vi "Synthetic_Jet_Per_Block.vi"() -> (5 "Plug in titles":string[](array[string]), 7 "Plug in values":string[](array[string]))   [LabVIEW 2011]
uses:
  Globals/Meas_global.vi
  Globals/Plug_in_data_global.vi
  Acquisition/Data_Translation/DataTranslation_global.vi
  <vilib>/Analysis/baseanly.llb/Scale 1D.vi
  <vilib>/Analysis/1siggen.llb/Ramp Pattern by Samples.vi
  <vilib>/Analysis/NI_AALBase.lvlib
panel:
  out "Pressure":cluster{dbl[], dbl[]}[](graph)=[{[0.0, 0.006711409395973154, 0.013422818791946308, 0.020134228187919462, 0.026845637583892617, 0.03355704697986577, 0.040268456375838924, 0.04697986577181208, 0.053691275167785234, 0.060402684563758385, 0.06711409395973154, 0.0738255033557047, 0.08053691275167785, 0.087248322147651, 0.09395973154362416, 0.10067114093959731, 0.10738255033557047, 0.11409395973154361, 0.12080536912751677, 0.12751677852348994, 0.1342281879194631, 0.14093959731543626, 0.1476510067114094, 0.15436241610738255, 0.1610738255033557, 0.16778523489932887, 0.174496644295302, 0.18120805369127518, 0.18791946308724833, 0.1946308724832215, 0.20134228187919462, 0.2080536912751678, 0.21476510067114093, 0.2214765100671141, 0.22818791946308722, 0.23489932885906042, 0.24161073825503354, 0.24832214765100674, 0.2550335570469799, 0.261744966442953, 0.2684563758389262, 0.2751677852348993, 0.2818791946308725, 0.2885906040268456, 0.2953020134228188, 0.30201342281879195, 0.3087248322147651, 0.31543624161073824, 0.3221476510067114, 0.3288590604026846, 0.33557046979865773, 0.3422818791946309, 0.348993288590604, 0.35570469798657717, 0.36241610738255037, 0.36912751677852346, 0.37583892617449666, 0.3825503355704698, 0.389261744966443, 0.3959731543624161, 0.40268456375838924, 0.40939597315436244, 0.4161073825503356, 0.4228187919463087, 0.42953020134228187, 0.436241610738255, 0.4429530201342282, 0.44966442953020136, 0.45637583892617445, 0.46308724832214765, 0.46979865771812085, 0.476510067114094, 0.4832214765100671, 0.4899328859060403, 0.4966442953020135, 0.5033557046979865, 0.5100671140939598, 0.5167785234899329, 0.523489932885906, 0.5302013422818792, 0.5369127516778524, 0.5436241610738255, 0.5503355704697986, 0.5570469798657718, 0.563758389261745, 0.5704697986577181, 0.5771812080536912, 0.5838926174496645, 0.5906040268456376, 0.5973154362416107, 0.6040268456375839, 0.610738255033557, 0.6174496644295302, 0.6241610738255033, 0.6308724832214765, 0.6375838926174497, 0.6442953020134228, 0.6510067114093959, 0.6577181208053692, 0.6644295302013422, 0.6711409395973155, 0.6778523489932886, 0.6845637583892618, 0.6912751677852349, 0.697986577181208, 0.7046979865771812, 0.7114093959731543, 0.7181208053691275, 0.7248322147651007, 0.7315436241610739, 0.7382550335570469, 0.7449664429530202, 0.7516778523489933, 0.7583892617449665, 0.7651006711409396, 0.7718120805369127, 0.778523489932886, 0.785234899328859, 0.7919463087248322, 0.7986577181208054, 0.8053691275167785, 0.8120805369127516, 0.8187919463087249, 0.825503355704698, 0.8322147651006712, 0.8389261744966443, 0.8456375838926175, 0.8523489932885906, 0.8590604026845637, 0.8657718120805369, 0.87248322147651, 0.8791946308724832, 0.8859060402684564, 0.8926174496644295, 0.8993288590604027, 0.9060402684563759, 0.9127516778523489, 0.9194630872483222, 0.9261744966442953, 0.9328859060402683, 0.9395973154362417, 0.9463087248322147, 0.953020134228188, 0.9597315436241611, 0.9664429530201342, 0.9731543624161074, 0.9798657718120806, 0.9865771812080536, 0.993288590604027, 1.0], [-0.25922546202362834, -0.4891204155324937, -0.6904080016618581, -0.8480493006444599, -0.9531546399067627, -0.9992739938596971, -0.9832658992629901, -0.9072023850623537, -0.7746259523585205, -0.5945933728335518, -0.3769969137121356, -0.13751047137392813, 0.11253663462306722, 0.35342670947288585, 0.5732288768268338, 0.7575057737083402, 0.8937918066214312, 0.975804049085562, 0.9976606124806482, 0.9561531939230075, 0.8553255918389477, 0.701995449856294, 0.5055203180524536, 0.2763271807993936, 0.030323873228706288, -0.21741726507064232, -0.4516233755794559, -0.6584586521118543, -0.8235859911563818, -0.9390514751472424, -0.9955643936504392, -0.9910192978985559, -0.924948310387722, -0.8008270925752599, -0.6293499874067777, -0.4169670204713452, -0.17941892779202917, 0.0689237672980099, 0.3128216261012807, 0.5372691486722271, 0.7283971090032636, 0.8738401730635315, 0.9660454611476949, 1.0, 0.9671483152639606, 0.8766808579084586, 0.7323072281427515, 0.5414132065636502, 0.3170325236361138, 0.0740370000188787, -0.17510777079208098, -0.41165326882024633, -0.6247046321897792, -0.7985879645210232, -0.9226089228683702, -0.9906182600380955, -0.9962662099062448, -0.9403548481937384, -0.826593775109834, -0.661900893747472, -0.4568702875871448, -0.22202920046593577, 0.02487644229078725, 0.27271784005525096, 0.5005073447966999, 0.6983526892904462, 0.8524849069940206, 0.954047745155591, 0.9966580178294975, 0.9763053464111373, 0.8967327509314734, 0.7603130387315623, 0.5771724157880267, 0.3585399421937547, 0.11718198984006566, -0.1316620025755488, -0.3727525963555975, -0.5900482770816685, -0.7717852675135934, -0.9053977146902825, -0.9835666776583354, -0.9990734749294669, -0.9541572345579136, -0.850889985489387, -0.6934157856153104, -0.4943673275401826, -0.26353661902357656, -0.017834089848234407, 0.23020782684645943, 0.4626092669832018, 0.6666372784923779, 0.8293249705524385, 0.9402453587914156, 0.993449714945815, 0.9842592639769333, 0.9139439591095612, 0.7875167735994525, 0.6119290303612525, 0.39834294984443913, 0.1592909651883969, -0.08865069204118191, -0.33274906977468277, -0.5549908841130975, -0.7432781595992073, -0.8855463405974977, -0.9741088681158134, -1.001914159774394, -0.9662217901934275, -0.8727465488844732, -0.723961502653703, -0.5304273151599044, -0.3054450754416776, -0.061246438243061585, 0.1873970352423227, 0.4244438305960635, 0.6338858532214537, 0.8049619205294755, 0.9253401183109746, 0.9892053975892771, 0.9910100679613483, 0.9305870303186635, 0.8139184327464221, 0.6452820124228671, 0.437343881774203, 0.20230227572276377, -0.045539122041699936, -0.2912416512170421, -0.519131415423606, -0.7137684570336703, -0.8649931502489075, -0.9626124494492849, -0.9992739938596971, -0.9772169115343806, -0.8929989608377183, -0.7531704268238946, -0.5669886001052015, -0.3462506777435128, -0.10325515412627774, 0.1451878004288764, 0.38474108241049404, 0.600633130624954, 0.7786605208476208, 0.9084965281716421, 0.9817527773490564, 0.9950538663876562, 0.9455925302642196, 0.83818122330427, 0.6770976826860506, 0.4746069829753056, 0.24411047267574976]}, {[0.0, 0.006711409395973154, 0.013422818791946308, 0.020134228187919462, 0.026845637583892617, 0.03355704697986577, 0.040268456375838924, 0.04697986577181208, 0.053691275167785234, 0.060402684563758385, 0.06711409395973154, 0.0738255033557047, 0.08053691275167785, 0.087248322147651, 0.09395973154362416, 0.10067114093959731, 0.10738255033557047, 0.11409395973154361, 0.12080536912751677, 0.12751677852348994, 0.1342281879194631, 0.14093959731543626, 0.1476510067114094, 0.15436241610738255, 0.1610738255033557, 0.16778523489932887, 0.174496644295302, 0.18120805369127518, 0.18791946308724833, 0.1946308724832215, 0.20134228187919462, 0.2080536912751678, 0.21476510067114093, 0.2214765100671141, 0.22818791946308722, 0.23489932885906042, 0.24161073825503354, 0.24832214765100674, 0.2550335570469799, 0.261744966442953, 0.2684563758389262, 0.2751677852348993, 0.2818791946308725, 0.2885906040268456, 0.2953020134228188, 0.30201342281879195, 0.3087248322147651, 0.31543624161073824, 0.3221476510067114, 0.3288590604026846, 0.33557046979865773, 0.3422818791946309, 0.348993288590604, 0.35570469798657717, 0.36241610738255037, 0.36912751677852346, 0.37583892617449666, 0.3825503355704698, 0.389261744966443, 0.3959731543624161, 0.40268456375838924, 0.40939597315436244, 0.4161073825503356, 0.4228187919463087, 0.42953020134228187, 0.436241610738255, 0.4429530201342282, 0.44966442953020136, 0.45637583892617445, 0.46308724832214765, 0.46979865771812085, 0.476510067114094, 0.4832214765100671, 0.4899328859060403, 0.4966442953020135, 0.5033557046979865, 0.5100671140939598, 0.5167785234899329, 0.523489932885906, 0.5302013422818792, 0.5369127516778524, 0.5436241610738255, 0.5503355704697986, 0.5570469798657718, 0.563758389261745, 0.5704697986577181, 0.5771812080536912, 0.5838926174496645, 0.5906040268456376, 0.5973154362416107, 0.6040268456375839, 0.610738255033557, 0.6174496644295302, 0.6241610738255033, 0.6308724832214765, 0.6375838926174497, 0.6442953020134228, 0.6510067114093959, 0.6577181208053692, 0.6644295302013422, 0.6711409395973155, 0.6778523489932886, 0.6845637583892618, 0.6912751677852349, 0.697986577181208, 0.7046979865771812, 0.7114093959731543, 0.7181208053691275, 0.7248322147651007, 0.7315436241610739, 0.7382550335570469, 0.7449664429530202, 0.7516778523489933, 0.7583892617449665, 0.7651006711409396, 0.7718120805369127, 0.778523489932886, 0.785234899328859, 0.7919463087248322, 0.7986577181208054, 0.8053691275167785, 0.8120805369127516, 0.8187919463087249, 0.825503355704698, 0.8322147651006712, 0.8389261744966443, 0.8456375838926175, 0.8523489932885906, 0.8590604026845637, 0.8657718120805369, 0.87248322147651, 0.8791946308724832, 0.8859060402684564, 0.8926174496644295, 0.8993288590604027, 0.9060402684563759, 0.9127516778523489, 0.9194630872483222, 0.9261744966442953, 0.9328859060402683, 0.9395973154362417, 0.9463087248322147, 0.953020134228188, 0.9597315436241611, 0.9664429530201342, 0.9731543624161074, 0.9798657718120806, 0.9865771812080536, 0.993288590604027, 1.0], [-0.06773154569815733, -0.3291387513527619, -0.5307198363636499, -0.7291484496532293, -0.8614105778258978, -0.9527614156827031, -1.0031655421930694, -0.9559138874040123, -0.8708679929898244, -0.7228435062106116, -0.5432943022183092, -0.27873462484239575, -0.09606837015936108, 0.17794872238047915, 0.4047141601312622, 0.6094477168634593, 0.7858444491344526, 0.8960746962885352, 0.9181065773071212, 0.9559008169322516, 0.9149541055858121, 0.7984189149891117, 0.6094477168634593, 0.4362388773443514, 0.2062855468416829, -0.026784834351717905, -0.25670274382380986, -0.4929255967385195, -0.6945066817494077, -0.8488361119712386, -0.9464564722400853, -1.0000130704717607, -0.9716408249799802, -0.9086622326149552, -0.7196910344893026, -0.5432943022183092, -0.3606280475352745, -0.11810025117794698, 0.127544595870113, 0.3700723922274406, 0.5874158358448734, 0.7826919774131437, 0.8866172811246085, 0.8740073942393727, 0.9685107038174874, 0.9307164641923568, 0.8078763301530385, 0.6818837243924114, 0.48660758282414107, 0.24407978646681344, 0.014161876994721509, -0.25039780038119197, -0.48031570985328387, -0.6724393797002453, -0.8299212816433852, -0.9275770629428083, -0.9874031835865249, -0.9905556553078338, -0.902357289172337, -0.7858220985756368, -0.5779714911527072, -0.38265992855386044, -0.12755766634187377, 0.039381650765192844, 0.33227815260231003, 0.5527740679410517, 0.7165254922962327, 0.8771598659606816, 0.9307164641923568, 1.0, 0.9338689359136656, 0.8519755132207868, 0.6944936112776469, 0.5023699414306856, 0.27245203195859363, 0.03622917904388393, -0.18111426457354876, -0.44252147022815336, -0.625187724911188, -0.7921270420182547, -0.8803254081537512, -0.9968605987504516, -0.9874031835865249, -0.8928998740084104, -0.7921270420182547, -0.625187724911188, -0.44567394194946225, -0.19684120214951692, 0.03622917904388393, 0.2944839129771795, 0.5180968790066537, 0.7039510264415737, 0.8614329283847134, 0.9464788227989014, 0.9622057603748693, 0.9716631755387962, 0.8677378718273314, 0.7259829074601595, 0.5275542941705804, 0.3385830960449279, 0.0866333055542501, -0.1558944908030775, -0.39211734371778717, -0.6063083156139111, -0.7795171551330188, -0.8897828233176781, -0.9433040005187766, -0.9968605987504516, -0.9275770629428083, -0.8299212816433852, -0.7102336193253758, -0.45513135711338903, -0.2126035607560615, 0.014161876994721509, 0.2503847299094312, 0.49291252626675885, 0.6724617302590611, 0.823638688759583, 0.9086491621431942, 0.9622057603748693, 0.9716631755387962, 0.8771598659606816, 0.7637771470852902, 0.5748059489596377, 0.3511929829301636, 0.10236024313021819, -0.11494777945663807, -0.3165288644675262, -0.5716665477100895, -0.7417229155078886, -0.8928998740084104, -1.0220449514903465, -0.9905556553078338, -0.9401515287974678, -0.8393786968073119, -0.7196910344893026, -0.5086525343144875, -0.3070714493035994, -0.03305435676375923, 0.20001602442964156, 0.4267814621804246, 0.6566993716525166, 0.8015713867104207, 0.9149541055858121, 0.9622057603748693, 0.9590532886535604, 0.8834648094032994, 0.8110288018743474, 0.634632069603354, 0.4047141601312622]}, {[0.0, 0.006711409395973154, 0.013422818791946308, 0.020134228187919462, 0.026845637583892617, 0.03355704697986577, 0.040268456375838924, 0.04697986577181208, 0.053691275167785234, 0.060402684563758385, 0.06711409395973154, 0.0738255033557047, 0.08053691275167785, 0.087248322147651, 0.09395973154362416, 0.10067114093959731, 0.10738255033557047, 0.11409395973154361, 0.12080536912751677, 0.12751677852348994, 0.1342281879194631, 0.14093959731543626, 0.1476510067114094, 0.15436241610738255, 0.1610738255033557, 0.16778523489932887, 0.174496644295302, 0.18120805369127518, 0.18791946308724833, 0.1946308724832215, 0.20134228187919462, 0.2080536912751678, 0.21476510067114093, 0.2214765100671141, 0.22818791946308722, 0.23489932885906042, 0.24161073825503354, 0.24832214765100674, 0.2550335570469799, 0.261744966442953, 0.2684563758389262, 0.2751677852348993, 0.2818791946308725, 0.2885906040268456, 0.2953020134228188, 0.30201342281879195, 0.3087248322147651, 0.31543624161073824, 0.3221476510067114, 0.3288590604026846, 0.33557046979865773, 0.3422818791946309, 0.348993288590604, 0.35570469798657717, 0.36241610738255037, 0.36912751677852346, 0.37583892617449666, 0.3825503355704698, 0.389261744966443, 0.3959731543624161, 0.40268456375838924, 0.40939597315436244, 0.4161073825503356, 0.4228187919463087, 0.42953020134228187, 0.436241610738255, 0.4429530201342282, 0.44966442953020136, 0.45637583892617445, 0.46308724832214765, 0.46979865771812085, 0.476510067114094, 0.4832214765100671, 0.4899328859060403, 0.4966442953020135, 0.5033557046979865, 0.5100671140939598, 0.5167785234899329, 0.523489932885906, 0.5302013422818792, 0.5369127516778524, 0.5436241610738255, 0.5503355704697986, 0.5570469798657718, 0.563758389261745, 0.5704697986577181, 0.5771812080536912, 0.5838926174496645, 0.5906040268456376, 0.5973154362416107, 0.6040268456375839, 0.610738255033557, 0.6174496644295302, 0.6241610738255033, 0.6308724832214765, 0.6375838926174497, 0.6442953020134228, 0.6510067114093959, 0.6577181208053692, 0.6644295302013422, 0.6711409395973155, 0.6778523489932886, 0.6845637583892618, 0.6912751677852349, 0.697986577181208, 0.7046979865771812, 0.7114093959731543, 0.7181208053691275, 0.7248322147651007, 0.7315436241610739, 0.7382550335570469, 0.7449664429530202, 0.7516778523489933, 0.7583892617449665, 0.7651006711409396, 0.7718120805369127, 0.778523489932886, 0.785234899328859, 0.7919463087248322, 0.7986577181208054, 0.8053691275167785, 0.8120805369127516, 0.8187919463087249, 0.825503355704698, 0.8322147651006712, 0.8389261744966443, 0.8456375838926175, 0.8523489932885906, 0.8590604026845637, 0.8657718120805369, 0.87248322147651, 0.8791946308724832, 0.8859060402684564, 0.8926174496644295, 0.8993288590604027, 0.9060402684563759, 0.9127516778523489, 0.9194630872483222, 0.9261744966442953, 0.9328859060402683, 0.9395973154362417, 0.9463087248322147, 0.953020134228188, 0.9597315436241611, 0.9664429530201342, 0.9731543624161074, 0.9798657718120806, 0.9865771812080536, 0.993288590604027, 1.0], [0.6373944760416457, 0.4107366158530138, 0.2092853682298436, -0.019859544398579457, -0.25407938835685134, -0.4807036397287289, -0.6620232061162826, -0.7980044787027606, -0.9012507637708912, -0.9264573763363528, -0.8937223888180068, -0.7829141199802374, -0.6771471736555602, -0.4781829784721823, -0.2641620333830344, -0.04758681822058906, 0.20172338446020602, 0.4157779383661059, 0.5794528759578378, 0.7658137648584848, 0.8967537149318688, 0.9521746537591312, 0.9496539925025853, 0.9118776824711464, 0.7985487523768298, 0.6499641735076223, 0.4560749096540908, 0.234458371978551, -0.002248524419510842, -0.23643475956102716, -0.4479686522103816, -0.6418915248806674, -0.7854347812367828, -0.8886810663049135, -0.8987301025143457, -0.8886810663049135, -0.82821880496456, -0.6871962098649912, -0.5109179659905284, -0.30442539585426615, -0.09037084194836505, 0.1664677356853132, 0.37548096707812095, 0.5265862072038764, 0.758251781088846, 0.8741013724397081, 0.9521746537591312, 0.9823889800209313, 0.9420920087329465, 0.816193381172654, 0.6927818060521538, 0.47620659088970607, 0.2747553432665359, 0.04308976938156619, -0.20117911078613437, -0.41019234217894335, -0.6015945535926824, -0.772831474954052, -0.8710364375090905, -0.9113334087970765, -0.8659951149959983, -0.8256981437080146, -0.6897168711215368, -0.5663389048177897, -0.3271113471631813, -0.11557745451382682, 0.11864238944444272, 0.34526664081632147, 0.5467178884394917, 0.7431614223663229, 0.8564567436438846, 0.9647443512251084, 0.9773476575078393, 0.9496539925025853, 0.8564567436438846, 0.702864451078338, 0.534148190973514, 0.3200936370676141, 0.10099776064861972, -0.14075045826253538, -0.3447223671422511, -0.5739008885874285, -0.7325345036660671, -0.8332601274776522, -0.8962094412577991, -0.8861604050483679, -0.8534254175300219, -0.7325345036660671, -0.5915119085664983, -0.3799780159171427, -0.16088213949815067, 0.08839445436589002, 0.32513495958070504, 0.5316275297169674, 0.7053851123348835, 0.8690600499266155, 0.9446126699894919, 0.9723063349947466, 0.9370506862198538, 0.8741013724397081, 0.7179548098008612, 0.5643625172353147, 0.3578699470990524, 0.10603908316171302, -0.12562649072325785, -0.3296320084197279, -0.5235212722732593, -0.7426171486922525, -0.82821880496456, -0.9239367150798062, -0.9339857512892373, -0.8659951149959983, -0.7602281686713211, -0.6217262348282977, -0.440406668440744, -0.20369977204268103, 0.02292447932919654, 0.26719335949689715, 0.4736859296331594, 0.657526157277261, 0.8388457236648147, 0.9118776824711464, 0.9723063349947466, 0.9672650124816545, 0.8892253399789851, 0.7658137648584848, 0.607180149779845, 0.4283812446488379, 0.1614264131722199, -0.07023916071274978, -0.30946671836735823, -0.54617361476542, -0.6746265123990136, -0.8206904300116756, -0.8937223888180068, -0.9289780375928997, -0.8811190825352758, -0.8030458012158527, -0.6368502023675753, -0.4656132810062046, -0.24903806584375807, -0.014851830702241725, 0.22689638820891336, 0.4409509421148133, 0.6323531535285536, 0.7960280911202844, 0.9068363599580538, 0.9849096412774775, 1.0, 0.9068363599580538]}]
  out "Displacement":cluster{dbl[], dbl[]}[](graph)=[{[0.0, 0.006711409395973154, 0.013422818791946308, 0.020134228187919462, 0.026845637583892617, 0.03355704697986577, 0.040268456375838924, 0.04697986577181208, 0.053691275167785234, 0.060402684563758385, 0.06711409395973154, 0.0738255033557047, 0.08053691275167785, 0.087248322147651, 0.09395973154362416, 0.10067114093959731, 0.10738255033557047, 0.11409395973154361, 0.12080536912751677, 0.12751677852348994, 0.1342281879194631, 0.14093959731543626, 0.1476510067114094, 0.15436241610738255, 0.1610738255033557, 0.16778523489932887, 0.174496644295302, 0.18120805369127518, 0.18791946308724833, 0.1946308724832215, 0.20134228187919462, 0.2080536912751678, 0.21476510067114093, 0.2214765100671141, 0.22818791946308722, 0.23489932885906042, 0.24161073825503354, 0.24832214765100674, 0.2550335570469799, 0.261744966442953, 0.2684563758389262, 0.2751677852348993, 0.2818791946308725, 0.2885906040268456, 0.2953020134228188, 0.30201342281879195, 0.3087248322147651, 0.31543624161073824, 0.3221476510067114, 0.3288590604026846, 0.33557046979865773, 0.3422818791946309, 0.348993288590604, 0.35570469798657717, 0.36241610738255037, 0.36912751677852346, 0.37583892617449666, 0.3825503355704698, 0.389261744966443, 0.3959731543624161, 0.40268456375838924, 0.40939597315436244, 0.4161073825503356, 0.4228187919463087, 0.42953020134228187, 0.436241610738255, 0.4429530201342282, 0.44966442953020136, 0.45637583892617445, 0.46308724832214765, 0.46979865771812085, 0.476510067114094, 0.4832214765100671, 0.4899328859060403, 0.4966442953020135, 0.5033557046979865, 0.5100671140939598, 0.5167785234899329, 0.523489932885906, 0.5302013422818792, 0.5369127516778524, 0.5436241610738255, 0.5503355704697986, 0.5570469798657718, 0.563758389261745, 0.5704697986577181, 0.5771812080536912, 0.5838926174496645, 0.5906040268456376, 0.5973154362416107, 0.6040268456375839, 0.610738255033557, 0.6174496644295302, 0.6241610738255033, 0.6308724832214765, 0.6375838926174497, 0.6442953020134228, 0.6510067114093959, 0.6577181208053692, 0.6644295302013422, 0.6711409395973155, 0.6778523489932886, 0.6845637583892618, 0.6912751677852349, 0.697986577181208, 0.7046979865771812, 0.7114093959731543, 0.7181208053691275, 0.7248322147651007, 0.7315436241610739, 0.7382550335570469, 0.7449664429530202, 0.7516778523489933, 0.7583892617449665, 0.7651006711409396, 0.7718120805369127, 0.778523489932886, 0.785234899328859, 0.7919463087248322, 0.7986577181208054, 0.8053691275167785, 0.8120805369127516, 0.8187919463087249, 0.825503355704698, 0.8322147651006712, 0.8389261744966443, 0.8456375838926175, 0.8523489932885906, 0.8590604026845637, 0.8657718120805369, 0.87248322147651, 0.8791946308724832, 0.8859060402684564, 0.8926174496644295, 0.8993288590604027, 0.9060402684563759, 0.9127516778523489, 0.9194630872483222, 0.9261744966442953, 0.9328859060402683, 0.9395973154362417, 0.9463087248322147, 0.953020134228188, 0.9597315436241611, 0.9664429530201342, 0.9731543624161074, 0.9798657718120806, 0.9865771812080536, 0.993288590604027, 1.0], [-0.25922546202362834, -0.4891204155324937, -0.6904080016618581, -0.8480493006444599, -0.9531546399067627, -0.9992739938596971, -0.9832658992629901, -0.9072023850623537, -0.7746259523585205, -0.5945933728335518, -0.3769969137121356, -0.13751047137392813, 0.11253663462306722, 0.35342670947288585, 0.5732288768268338, 0.7575057737083402, 0.8937918066214312, 0.975804049085562, 0.9976606124806482, 0.9561531939230075, 0.8553255918389477, 0.701995449856294, 0.5055203180524536, 0.2763271807993936, 0.030323873228706288, -0.21741726507064232, -0.4516233755794559, -0.6584586521118543, -0.8235859911563818, -0.9390514751472424, -0.9955643936504392, -0.9910192978985559, -0.924948310387722, -0.8008270925752599, -0.6293499874067777, -0.4169670204713452, -0.17941892779202917, 0.0689237672980099, 0.3128216261012807, 0.5372691486722271, 0.7283971090032636, 0.8738401730635315, 0.9660454611476949, 1.0, 0.9671483152639606, 0.8766808579084586, 0.7323072281427515, 0.5414132065636502, 0.3170325236361138, 0.0740370000188787, -0.17510777079208098, -0.41165326882024633, -0.6247046321897792, -0.7985879645210232, -0.9226089228683702, -0.9906182600380955, -0.9962662099062448, -0.9403548481937384, -0.826593775109834, -0.661900893747472, -0.4568702875871448, -0.22202920046593577, 0.02487644229078725, 0.27271784005525096, 0.5005073447966999, 0.6983526892904462, 0.8524849069940206, 0.954047745155591, 0.9966580178294975, 0.9763053464111373, 0.8967327509314734, 0.7603130387315623, 0.5771724157880267, 0.3585399421937547, 0.11718198984006566, -0.1316620025755488, -0.3727525963555975, -0.5900482770816685, -0.7717852675135934, -0.9053977146902825, -0.9835666776583354, -0.9990734749294669, -0.9541572345579136, -0.850889985489387, -0.6934157856153104, -0.4943673275401826, -0.26353661902357656, -0.017834089848234407, 0.23020782684645943, 0.4626092669832018, 0.6666372784923779, 0.8293249705524385, 0.9402453587914156, 0.993449714945815, 0.9842592639769333, 0.9139439591095612, 0.7875167735994525, 0.6119290303612525, 0.39834294984443913, 0.1592909651883969, -0.08865069204118191, -0.33274906977468277, -0.5549908841130975, -0.7432781595992073, -0.8855463405974977, -0.9741088681158134, -1.001914159774394, -0.9662217901934275, -0.8727465488844732, -0.723961502653703, -0.5304273151599044, -0.3054450754416776, -0.061246438243061585, 0.1873970352423227, 0.4244438305960635, 0.6338858532214537, 0.8049619205294755, 0.9253401183109746, 0.9892053975892771, 0.9910100679613483, 0.9305870303186635, 0.8139184327464221, 0.6452820124228671, 0.437343881774203, 0.20230227572276377, -0.045539122041699936, -0.2912416512170421, -0.519131415423606, -0.7137684570336703, -0.8649931502489075, -0.9626124494492849, -0.9992739938596971, -0.9772169115343806, -0.8929989608377183, -0.7531704268238946, -0.5669886001052015, -0.3462506777435128, -0.10325515412627774, 0.1451878004288764, 0.38474108241049404, 0.600633130624954, 0.7786605208476208, 0.9084965281716421, 0.9817527773490564, 0.9950538663876562, 0.9455925302642196, 0.83818122330427, 0.6770976826860506, 0.4746069829753056, 0.24411047267574976]}, {[0.0, 0.006711409395973154, 0.013422818791946308, 0.020134228187919462, 0.026845637583892617, 0.03355704697986577, 0.040268456375838924, 0.04697986577181208, 0.053691275167785234, 0.060402684563758385, 0.06711409395973154, 0.0738255033557047, 0.08053691275167785, 0.087248322147651, 0.09395973154362416, 0.10067114093959731, 0.10738255033557047, 0.11409395973154361, 0.12080536912751677, 0.12751677852348994, 0.1342281879194631, 0.14093959731543626, 0.1476510067114094, 0.15436241610738255, 0.1610738255033557, 0.16778523489932887, 0.174496644295302, 0.18120805369127518, 0.18791946308724833, 0.1946308724832215, 0.20134228187919462, 0.2080536912751678, 0.21476510067114093, 0.2214765100671141, 0.22818791946308722, 0.23489932885906042, 0.24161073825503354, 0.24832214765100674, 0.2550335570469799, 0.261744966442953, 0.2684563758389262, 0.2751677852348993, 0.2818791946308725, 0.2885906040268456, 0.2953020134228188, 0.30201342281879195, 0.3087248322147651, 0.31543624161073824, 0.3221476510067114, 0.3288590604026846, 0.33557046979865773, 0.3422818791946309, 0.348993288590604, 0.35570469798657717, 0.36241610738255037, 0.36912751677852346, 0.37583892617449666, 0.3825503355704698, 0.389261744966443, 0.3959731543624161, 0.40268456375838924, 0.40939597315436244, 0.4161073825503356, 0.4228187919463087, 0.42953020134228187, 0.436241610738255, 0.4429530201342282, 0.44966442953020136, 0.45637583892617445, 0.46308724832214765, 0.46979865771812085, 0.476510067114094, 0.4832214765100671, 0.4899328859060403, 0.4966442953020135, 0.5033557046979865, 0.5100671140939598, 0.5167785234899329, 0.523489932885906, 0.5302013422818792, 0.5369127516778524, 0.5436241610738255, 0.5503355704697986, 0.5570469798657718, 0.563758389261745, 0.5704697986577181, 0.5771812080536912, 0.5838926174496645, 0.5906040268456376, 0.5973154362416107, 0.6040268456375839, 0.610738255033557, 0.6174496644295302, 0.6241610738255033, 0.6308724832214765, 0.6375838926174497, 0.6442953020134228, 0.6510067114093959, 0.6577181208053692, 0.6644295302013422, 0.6711409395973155, 0.6778523489932886, 0.6845637583892618, 0.6912751677852349, 0.697986577181208, 0.7046979865771812, 0.7114093959731543, 0.7181208053691275, 0.7248322147651007, 0.7315436241610739, 0.7382550335570469, 0.7449664429530202, 0.7516778523489933, 0.7583892617449665, 0.7651006711409396, 0.7718120805369127, 0.778523489932886, 0.785234899328859, 0.7919463087248322, 0.7986577181208054, 0.8053691275167785, 0.8120805369127516, 0.8187919463087249, 0.825503355704698, 0.8322147651006712, 0.8389261744966443, 0.8456375838926175, 0.8523489932885906, 0.8590604026845637, 0.8657718120805369, 0.87248322147651, 0.8791946308724832, 0.8859060402684564, 0.8926174496644295, 0.8993288590604027, 0.9060402684563759, 0.9127516778523489, 0.9194630872483222, 0.9261744966442953, 0.9328859060402683, 0.9395973154362417, 0.9463087248322147, 0.953020134228188, 0.9597315436241611, 0.9664429530201342, 0.9731543624161074, 0.9798657718120806, 0.9865771812080536, 0.993288590604027, 1.0], [-1.8900299638896667, -0.3337772428099433, -1.6677337567546753, -1.445437549619689, -1.3342894460521906, -1.1118139677824157, -1.3342894460521906, -2.5569185852946408, -1.6677337567546753, -3.6683996209695926, -3.4461034138346065, -4.780059927779338, -4.224319409941858, -5.113504238481823, -5.558096652751805, -4.557763720644347, -5.891540963454291, -4.335467513509355, -2.668066688862134, -4.1131713063743645, -3.3349553102671083, -3.4461034138346065, -2.5569185852946408, -2.5569185852946408, -1.7788818603221734, -2.4457704817271475, -0.8895177606474244, -1.1118139677824157, -1.2231413424846975, -1.445437549619689, -2.0011780674571646, -0.8895177606474244, -3.4461034138346065, -1.8900299638896667, -3.890695828104584, -4.66891182421184, -4.1131713063743645, -4.335467513509355, -4.891208031346832, -5.446948549184308, -5.002356134914325, -5.780392859886797, -4.557763720644347, -1.6677337567546753, -4.557763720644347, -3.5572515174020998, -4.446615617076849, -2.5569185852946408, -3.5572515174020998, -1.7788818603221734, -1.8900299638896667, -0.667221553512433, -0.4449253463774415, -1.445437549619689, -0.667221553512433, -2.3346223781596493, -1.8900299638896667, -1.556585653187182, -3.0015109995646236, -3.112659103132117, -4.780059927779338, -4.891208031346832, -6.1138371705892816, -3.0015109995646236, -4.1131713063743645, -5.224652342049316, -5.558096652751805, -5.224652342049316, -4.446615617076849, -5.446948549184308, -2.8903628959971255, -4.002023202806866, -3.5572515174020998, -1.6677337567546753, -2.0011780674571646, -1.6677337567546753, -1.556585653187182, -0.22262913924245015, -1.7788818603221734, -1.1118139677824157, -2.4457704817271475, -1.556585653187182, -1.8900299638896667, -3.3349553102671083, -2.4457704817271475, -4.891208031346832, -3.223807206699615, -5.002356134914325, -4.557763720644347, -5.335800445616814, -5.891540963454291, -5.113504238481823, -6.1138371705892816, -4.1131713063743645, -4.780059927779338, -5.224652342049316, -3.3349553102671083, -2.779214792429632, -2.3346223781596493, -2.112326171024658, -0.8895177606474244, -2.0011780674571646, -1.445437549619689, -0.8895177606474244, -0.8895177606474244, -1.8900299638896667, -2.668066688862134, -0.5560734499449347, -3.6683996209695926, -2.5569185852946408, -1.2231413424846975, -5.335800445616814, -5.002356134914325, -4.780059927779338, -4.446615617076849, -5.558096652751805, -5.002356134914325, -5.335800445616814, -4.557763720644347, -3.890695828104584, -5.002356134914325, -3.223807206699615, -4.002023202806866, -2.4457704817271475, -2.112326171024658, -1.3342894460521906, -1.445437549619689, -2.112326171024658, -1.0006658642149175, -1.1118139677824157, -0.667221553512433, 1.0, -2.4457704817271475, -1.8900299638896667, -3.4461034138346065, -2.8903628959971255, -3.5572515174020998, -3.890695828104584, -5.224652342049316, -4.446615617076849, -4.1131713063743645, -5.558096652751805, -4.780059927779338, -5.446948549184308, -4.335467513509355, -5.002356134914325, -2.5569185852946408, -4.335467513509355, -5.558096652751805, -1.7788818603221734]}]
  out "Hot Wire":cluster{dbl[], dbl[]}[](graph)=[{[0.0, 0.006711409395973154, 0.013422818791946308, 0.020134228187919462, 0.026845637583892617, 0.03355704697986577, 0.040268456375838924, 0.04697986577181208, 0.053691275167785234, 0.060402684563758385, 0.06711409395973154, 0.0738255033557047, 0.08053691275167785, 0.087248322147651, 0.09395973154362416, 0.10067114093959731, 0.10738255033557047, 0.11409395973154361, 0.12080536912751677, 0.12751677852348994, 0.1342281879194631, 0.14093959731543626, 0.1476510067114094, 0.15436241610738255, 0.1610738255033557, 0.16778523489932887, 0.174496644295302, 0.18120805369127518, 0.18791946308724833, 0.1946308724832215, 0.20134228187919462, 0.2080536912751678, 0.21476510067114093, 0.2214765100671141, 0.22818791946308722, 0.23489932885906042, 0.24161073825503354, 0.24832214765100674, 0.2550335570469799, 0.261744966442953, 0.2684563758389262, 0.2751677852348993, 0.2818791946308725, 0.2885906040268456, 0.2953020134228188, 0.30201342281879195, 0.3087248322147651, 0.31543624161073824, 0.3221476510067114, 0.3288590604026846, 0.33557046979865773, 0.3422818791946309, 0.348993288590604, 0.35570469798657717, 0.36241610738255037, 0.36912751677852346, 0.37583892617449666, 0.3825503355704698, 0.389261744966443, 0.3959731543624161, 0.40268456375838924, 0.40939597315436244, 0.4161073825503356, 0.4228187919463087, 0.42953020134228187, 0.436241610738255, 0.4429530201342282, 0.44966442953020136, 0.45637583892617445, 0.46308724832214765, 0.46979865771812085, 0.476510067114094, 0.4832214765100671, 0.4899328859060403, 0.4966442953020135, 0.5033557046979865, 0.5100671140939598, 0.5167785234899329, 0.523489932885906, 0.5302013422818792, 0.5369127516778524, 0.5436241610738255, 0.5503355704697986, 0.5570469798657718, 0.563758389261745, 0.5704697986577181, 0.5771812080536912, 0.5838926174496645, 0.5906040268456376, 0.5973154362416107, 0.6040268456375839, 0.610738255033557, 0.6174496644295302, 0.6241610738255033, 0.6308724832214765, 0.6375838926174497, 0.6442953020134228, 0.6510067114093959, 0.6577181208053692, 0.6644295302013422, 0.6711409395973155, 0.6778523489932886, 0.6845637583892618, 0.6912751677852349, 0.697986577181208, 0.7046979865771812, 0.7114093959731543, 0.7181208053691275, 0.7248322147651007, 0.7315436241610739, 0.7382550335570469, 0.7449664429530202, 0.7516778523489933, 0.7583892617449665, 0.7651006711409396, 0.7718120805369127, 0.778523489932886, 0.785234899328859, 0.7919463087248322, 0.7986577181208054, 0.8053691275167785, 0.8120805369127516, 0.8187919463087249, 0.825503355704698, 0.8322147651006712, 0.8389261744966443, 0.8456375838926175, 0.8523489932885906, 0.8590604026845637, 0.8657718120805369, 0.87248322147651, 0.8791946308724832, 0.8859060402684564, 0.8926174496644295, 0.8993288590604027, 0.9060402684563759, 0.9127516778523489, 0.9194630872483222, 0.9261744966442953, 0.9328859060402683, 0.9395973154362417, 0.9463087248322147, 0.953020134228188, 0.9597315436241611, 0.9664429530201342, 0.9731543624161074, 0.9798657718120806, 0.9865771812080536, 0.993288590604027, 1.0], [-0.25922546202362834, -0.4891204155324937, -0.6904080016618581, -0.8480493006444599, -0.9531546399067627, -0.9992739938596971, -0.9832658992629901, -0.9072023850623537, -0.7746259523585205, -0.5945933728335518, -0.3769969137121356, -0.13751047137392813, 0.11253663462306722, 0.35342670947288585, 0.5732288768268338, 0.7575057737083402, 0.8937918066214312, 0.975804049085562, 0.9976606124806482, 0.9561531939230075, 0.8553255918389477, 0.701995449856294, 0.5055203180524536, 0.2763271807993936, 0.030323873228706288, -0.21741726507064232, -0.4516233755794559, -0.6584586521118543, -0.8235859911563818, -0.9390514751472424, -0.9955643936504392, -0.9910192978985559, -0.924948310387722, -0.8008270925752599, -0.6293499874067777, -0.4169670204713452, -0.17941892779202917, 0.0689237672980099, 0.3128216261012807, 0.5372691486722271, 0.7283971090032636, 0.8738401730635315, 0.9660454611476949, 1.0, 0.9671483152639606, 0.8766808579084586, 0.7323072281427515, 0.5414132065636502, 0.3170325236361138, 0.0740370000188787, -0.17510777079208098, -0.41165326882024633, -0.6247046321897792, -0.7985879645210232, -0.9226089228683702, -0.9906182600380955, -0.9962662099062448, -0.9403548481937384, -0.826593775109834, -0.661900893747472, -0.4568702875871448, -0.22202920046593577, 0.02487644229078725, 0.27271784005525096, 0.5005073447966999, 0.6983526892904462, 0.8524849069940206, 0.954047745155591, 0.9966580178294975, 0.9763053464111373, 0.8967327509314734, 0.7603130387315623, 0.5771724157880267, 0.3585399421937547, 0.11718198984006566, -0.1316620025755488, -0.3727525963555975, -0.5900482770816685, -0.7717852675135934, -0.9053977146902825, -0.9835666776583354, -0.9990734749294669, -0.9541572345579136, -0.850889985489387, -0.6934157856153104, -0.4943673275401826, -0.26353661902357656, -0.017834089848234407, 0.23020782684645943, 0.4626092669832018, 0.6666372784923779, 0.8293249705524385, 0.9402453587914156, 0.993449714945815, 0.9842592639769333, 0.9139439591095612, 0.7875167735994525, 0.6119290303612525, 0.39834294984443913, 0.1592909651883969, -0.08865069204118191, -0.33274906977468277, -0.5549908841130975, -0.7432781595992073, -0.8855463405974977, -0.9741088681158134, -1.001914159774394, -0.9662217901934275, -0.8727465488844732, -0.723961502653703, -0.5304273151599044, -0.3054450754416776, -0.061246438243061585, 0.1873970352423227, 0.4244438305960635, 0.6338858532214537, 0.8049619205294755, 0.9253401183109746, 0.9892053975892771, 0.9910100679613483, 0.9305870303186635, 0.8139184327464221, 0.6452820124228671, 0.437343881774203, 0.20230227572276377, -0.045539122041699936, -0.2912416512170421, -0.519131415423606, -0.7137684570336703, -0.8649931502489075, -0.9626124494492849, -0.9992739938596971, -0.9772169115343806, -0.8929989608377183, -0.7531704268238946, -0.5669886001052015, -0.3462506777435128, -0.10325515412627774, 0.1451878004288764, 0.38474108241049404, 0.600633130624954, 0.7786605208476208, 0.9084965281716421, 0.9817527773490564, 0.9950538663876562, 0.9455925302642196, 0.83818122330427, 0.6770976826860506, 0.4746069829753056, 0.24411047267574976]}, {[0.0, 0.006711409395973154, 0.013422818791946308, 0.020134228187919462, 0.026845637583892617, 0.03355704697986577, 0.040268456375838924, 0.04697986577181208, 0.053691275167785234, 0.060402684563758385, 0.06711409395973154, 0.0738255033557047, 0.08053691275167785, 0.087248322147651, 0.09395973154362416, 0.10067114093959731, 0.10738255033557047, 0.11409395973154361, 0.12080536912751677, 0.12751677852348994, 0.1342281879194631, 0.14093959731543626, 0.1476510067114094, 0.15436241610738255, 0.1610738255033557, 0.16778523489932887, 0.174496644295302, 0.18120805369127518, 0.18791946308724833, 0.1946308724832215, 0.20134228187919462, 0.2080536912751678, 0.21476510067114093, 0.2214765100671141, 0.22818791946308722, 0.23489932885906042, 0.24161073825503354, 0.24832214765100674, 0.2550335570469799, 0.261744966442953, 0.2684563758389262, 0.2751677852348993, 0.2818791946308725, 0.2885906040268456, 0.2953020134228188, 0.30201342281879195, 0.3087248322147651, 0.31543624161073824, 0.3221476510067114, 0.3288590604026846, 0.33557046979865773, 0.3422818791946309, 0.348993288590604, 0.35570469798657717, 0.36241610738255037, 0.36912751677852346, 0.37583892617449666, 0.3825503355704698, 0.389261744966443, 0.3959731543624161, 0.40268456375838924, 0.40939597315436244, 0.4161073825503356, 0.4228187919463087, 0.42953020134228187, 0.436241610738255, 0.4429530201342282, 0.44966442953020136, 0.45637583892617445, 0.46308724832214765, 0.46979865771812085, 0.476510067114094, 0.4832214765100671, 0.4899328859060403, 0.4966442953020135, 0.5033557046979865, 0.5100671140939598, 0.5167785234899329, 0.523489932885906, 0.5302013422818792, 0.5369127516778524, 0.5436241610738255, 0.5503355704697986, 0.5570469798657718, 0.563758389261745, 0.5704697986577181, 0.5771812080536912, 0.5838926174496645, 0.5906040268456376, 0.5973154362416107, 0.6040268456375839, 0.610738255033557, 0.6174496644295302, 0.6241610738255033, 0.6308724832214765, 0.6375838926174497, 0.6442953020134228, 0.6510067114093959, 0.6577181208053692, 0.6644295302013422, 0.6711409395973155, 0.6778523489932886, 0.6845637583892618, 0.6912751677852349, 0.697986577181208, 0.7046979865771812, 0.7114093959731543, 0.7181208053691275, 0.7248322147651007, 0.7315436241610739, 0.7382550335570469, 0.7449664429530202, 0.7516778523489933, 0.7583892617449665, 0.7651006711409396, 0.7718120805369127, 0.778523489932886, 0.785234899328859, 0.7919463087248322, 0.7986577181208054, 0.8053691275167785, 0.8120805369127516, 0.8187919463087249, 0.825503355704698, 0.8322147651006712, 0.8389261744966443, 0.8456375838926175, 0.8523489932885906, 0.8590604026845637, 0.8657718120805369, 0.87248322147651, 0.8791946308724832, 0.8859060402684564, 0.8926174496644295, 0.8993288590604027, 0.9060402684563759, 0.9127516778523489, 0.9194630872483222, 0.9261744966442953, 0.9328859060402683, 0.9395973154362417, 0.9463087248322147, 0.953020134228188, 0.9597315436241611, 0.9664429530201342, 0.9731543624161074, 0.9798657718120806, 0.9865771812080536, 0.993288590604027, 1.0], [0.786162494909381, 0.9555541396592179, 0.9801114006514251, 0.938564221627578, 0.7795777785761965, 0.6615088292662319, 0.505575171149091, 0.3563258510797405, 0.3187398245784116, 0.27995335246102476, 0.33208211467880283, 0.4215723550703854, 0.5510362905126058, 0.5037872511325407, 0.552898894986484, 0.4722062752500574, 0.39878683517833774, 0.34716040156338873, 0.23373435457518954, 0.15789284363450184, 0.1781396982954223, 0.20535857404616356, 0.31433499800077797, 0.4670263324025916, 0.6216623195914813, 0.7256727991271182, 0.9677914605148665, 1.0, 0.9751776162981031, 0.8422612429410716, 0.6021770469769608, 0.4722062752500574, 0.41011305544034105, 0.3172648643903663, 0.2941020442865551, 0.3350743124071423, 0.36404278994568134, 0.4739433477686833, 0.549192080984425, 0.5547644111207934, 0.5145275905899821, 0.41992124486815724, 0.3172648643903663, 0.2729741416193657, 0.20915200786852417, 0.17451497490363752, 0.19907025559403857, 0.2743695855932228, 0.405238838821954, 0.641427842131357, 0.7708113771183738, 0.8537192754068978, 0.9751776162981031, 0.9801114006514251, 0.8399715922584555, 0.7448480520398097, 0.5289874633694818, 0.40848106967981207, 0.32760714155264725, 0.3055951519532317, 0.33208211467880283, 0.39878683517833774, 0.4381650866696267, 0.5436457719645258, 0.5622243250514745, 0.5145275905899821, 0.4248690125191858, 0.3718261099722829, 0.2605748818963137, 0.20031681410189425, 0.18299903311750762, 0.19907025559403857, 0.28840491947472346, 0.3502050192728885, 0.5547644111207934, 0.7883759510791727, 0.905065445751601, 0.9801114006514251, 0.9506863527044238, 0.8722031919612652, 0.710929089712886, 0.6002383102800514, 0.44320344710272985, 0.3261165635377511, 0.32020506939924526, 0.31433499800077797, 0.36404278994568134, 0.45675605165331007, 0.47914236125078713, 0.5547644111207934, 0.5235511963000332, 0.4314951266336146, 0.3441136202794757, 0.2855775854712253, 0.2129778104599778, 0.1602379487289258, 0.18299903311750762, 0.24703051874683812, 0.3859989102248488, 0.5829865535730815, 0.6963354011857562, 0.8885551203925042, 0.9169587702814905, 0.9776531763255869, 0.9900394879119553, 0.7362988230396326, 0.5640887038837356, 0.5109410919058975, 0.34716040156338873, 0.2813614841852256, 0.3395884949164165, 0.3305836878895049, 0.4381650866696267, 0.5584885803940975, 0.5145275905899821, 0.541797645110199, 0.46359178766955267, 0.3828321414508846, 0.31433499800077797, 0.22588143497341914, 0.16496604715069035, 0.1757242130459757, 0.2363826785369679, 0.3305836878895049, 0.516317576006603, 0.6818910012134328, 0.8354209341672979, 0.9974944539227906, 0.9702570546079078, 0.8909124482457045, 0.8263577563423137, 0.6216623195914813, 0.4808906680350603, 0.3578690897371822, 0.2743695855932228, 0.3027065123004718, 0.3718261099722829, 0.4722062752500574, 0.47741141203471454, 0.5344646890699905, 0.5271775911041975, 0.46016836643378256, 0.3907758436880671, 0.29267094790431386, 0.23902983136949368, 0.16496604715069035, 0.17451497490363752, 0.19532403308345303, 0.3027065123004718, 0.4861378995500955]}]
  out "Input Voltage":dbl[](array[numeric])=[-0.784562842644, -1.48410152415, -2.0938495778970005, -2.5722952513440003, -2.8909560281490005, -3.0276115054920005, -2.9797366375980006, -2.7469274171430005, -2.3382740089170007, -1.785894995178, -1.125141016776, -0.393685756674, 0.363120963009, 1.095586241421, 1.758764263767, 2.31356732145, 2.7218167223519996, 2.9632110984419997, 3.0172470780269998, 2.8833186501209997, 2.5726370179649996, 2.0974234031099996, 1.49444247204, 0.7953077978580001, 0.044561188035000004, -0.7046703943229999, -1.410168183858, -2.0306224316910004, -2.5250263944360003, -2.8640895411030005, -3.0209453846460006, -2.9910488426700006, -2.7777329755980005, -2.3907949610370003, -1.854879245751, -1.202104411998, -0.478224289221, 0.276764397504, 1.0155927912690002, 1.6903860241800002, 2.257713308907, 2.6831330210789996, 2.9422027175939998, 3.0190651109849997, 2.908670109702, 2.6144517759989996, 2.157317488893, 1.567062788529, 0.878634308433, 0.135159830442, -0.619828856283, -1.334214806946, -1.964769237879, -2.4749294862600006, -2.8323749661690005, -3.0117542180250005, -3.0047850916860006, -2.8115685889830004, -2.4471539827350006, -1.922954479845, -1.282703873136, -0.56397484374, 0.18949881552, 0.9328722916800001, 1.6165536857190002, 2.200041263406, 2.6431362960029996, 2.922709364211, 3.0205801384499997, 2.9317995290009997, 2.6553575175539996, 2.215292539887, 1.639986110511, 0.9600417842190001, 0.219698362989, -0.534078301764, -1.256140391583, -1.900330069701, -2.4258425963940007, -2.8027814296860005, -3.0004420129530005, -3.0138752564760005, -2.8414651309590004, -2.4917967920370003, -1.989716690136, -1.358051239062, -0.6460893323429999, 0.110818389171, 0.850858804908, 1.5435293619060002, 2.1374201281859997, 2.5998065105039996, 2.8988729320949997, 3.0190651109849997, 2.951696889708, 2.6953542426299997, 2.272661579895, 1.7074553336190001, 1.0409442508500002, 0.303024873564, -0.45135780217500004, -1.178267979882, -1.830739808142, -2.3708976003300006, -2.7661177650330004, -2.9889278042190006, -3.0233694285900006, -2.8704526564560005, -2.5396716599310003, -2.0505197923980005, -1.431883577523, -0.729415842918, 0.021633772398000004, 0.77025934377, 1.4693940179520002, 2.0782330552199997, 2.5546586920469996, 2.8753395054719997, 3.015429045069, 2.967857182668, 2.7316138999589996, 2.330636630889, 1.7779546116570002, 1.120634695509, 0.389381439069, -0.36712227512100004, -1.099587553533, -1.763270585034, -2.3192856646890005, -2.7303631168590003, -2.9726665094280005, -3.0294295384500005, -2.8973191435020005, -2.5863345058530003, -2.1136459367730005, -1.509654987393, -0.812035340676, -0.06532880409300001, 0.6854178057300001, 1.3934406410400002, 2.0157129218309997, 2.5095108735899996, 2.8481700129329997, 3.009974946195, 2.981896437177, 2.7691865810909997, 2.3837635939949995, 1.8493629061740002, 1.199012116365, 0.474222977109]
  out "Displacement":dbl[](array[numeric])=[-0.009780325190983985, -0.001846017406867989, -0.007339133946211968, -0.011611654863169979, -0.01100092081336998, -0.009169591141183986, -0.018935228597485976, -0.024428345136829982, -0.017104771402513985, -0.018935228597485976, -0.02015582421987197, -0.02015582421987197, -0.026870408858815975, -0.02503907918662998, -0.02503907918662998, -0.023818483564243986, -0.029921461676173988, -0.02503907918662998, -0.023818483564243986, -0.026870408858815975, -0.02015582421987197, -0.01832536702489998, -0.01344211205814197, -0.01344211205814197, -0.01832536702489998, -0.014662707680527992, -0.007339133946211968, -0.0048970702242259745, -0.0067283998964119685, -0.017104771402513985, -0.009780325190983985, -0.005507804274025974, -0.01588417578012799, -0.01832536702489998, -0.021987153892057992, -0.019545962647285975, -0.02015582421987197, -0.024428345136829982, -0.026870408858815975, -0.021987153892057992, -0.023818483564243986, -0.028700866053787993, -0.03175279134835998, -0.028700866053787993, -0.02015582421987197, -0.023207749514443987, -0.02503907918662998, -0.01344211205814197, -0.01039018676356998, -0.007948995518797991, -0.01100092081336998, -0.009169591141183986, -0.002455878979453985, -0.005507804274025974, -0.007948995518797991, -0.00855972956859799, -0.01100092081336998, -0.012832250485555974, -0.029311600103587993, -0.02503907918662998, -0.02076655826967197, -0.019545962647285975, -0.029311600103587993, -0.02748027043140197, -0.026259674809015976, -0.023207749514443987, -0.028700866053787993, -0.03297338697074598, -0.031142929775773986, -0.018935228597485976, -0.026259674809015976, -0.024428345136829982, -0.01771463297509998, -0.014052846107941969, -0.006118538323825973, -0.009780325190983985, -0.00855972956859799, -0.006118538323825973, -0.0048970702242259745, -0.009780325190983985, -0.01039018676356998, -0.0067283998964119685, -0.007948995518797991, -0.014052846107941969, -0.02259788794185799, -0.015273441730327991, -0.021987153892057992, -0.016494037352713986, -0.029311600103587993, -0.02748027043140197, -0.029311600103587993, -0.030532195725973987, -0.03419398259313197, -0.02748027043140197, -0.02137729231947197, -0.023207749514443987, -0.02503907918662998, -0.030532195725973987, -0.01039018676356998, -0.01344211205814197, -0.01344211205814197, -0.01039018676356998, -0.003066613029253984, -0.003066613029253984, -0.0067283998964119685, -0.012221516435755975, -0.01100092081336998, -0.011611654863169979, -0.014052846107941969, -0.02137729231947197, -0.01588417578012799, -0.017104771402513985, -0.02015582421987197, -0.028700866053787993, -0.028700866053787993, -0.02503907918662998, -0.029921461676173988, -0.02809100448120197, -0.026259674809015976, -0.02259788794185799, -0.02748027043140197, -0.02259788794185799, -0.02564981323642998, -0.015273441730327991, -0.007339133946211968, -0.012221516435755975, -0.01100092081336998, -0.007339133946211968, -0.005507804274025974, -0.0067283998964119685, -0.01344211205814197, -0.01588417578012799, -0.009169591141183986, -0.01771463297509998, -0.02015582421987197, -0.01771463297509998, -0.024428345136829982, -0.023207749514443987, -0.02748027043140197, -0.029921461676173988, -0.02748027043140197, -0.02748027043140197, -0.02809100448120197, -0.026259674809015976, -0.026870408858815975, -0.019545962647285975, -0.019545962647285975, -0.023207749514443987, -0.014052846107941969, -0.011611654863169979]
  out "Honey Pressure":dbl[](array[numeric])=[-14.369666524328046, -57.77058962565634, -87.07652966541758, -117.51006835010423, -142.3114261743131, -158.09199483911908, -155.83679754926837, -151.8902022920296, -142.3114261743131, -120.32906496241762, -88.20412831034297, -49.31359978871612, -12.114469234477319, 29.02544421285115, 67.35217341201532, 101.7323073539407, 128.78305010385122, 147.3826153809706, 157.5310031852989, 162.59938472331393, 149.63781267082135, 136.11244129586606, 102.29610667640338, 72.99016663664214, 42.55081558780641, -5.354689729074237, -48.18600114379076, -84.25753305310417, -116.38246970517886, -138.36483091707433, -158.65579416158175, -165.41557366698484, -160.34719212896982, -149.0712056797162, -122.58426225226835, -92.71452289004439, -56.642990980730964, -17.188663136641456, 24.515049633149694, 61.15038086492581, 97.22191277423924, 132.1658460386273, 151.3292106382094, 160.34418743346322, 160.34418743346322, 155.27580589544817, 136.67624061832876, 106.80650125610484, 74.67575223988108, 33.5358387925526, -1.9718937942981463, -42.553820283313044, -85.38513169802953, -116.38246970517886, -141.74762685185044, -159.78339280650712, -164.28797502205947, -162.03859009635784, -141.18382752938774, -123.71186089719372, -94.40592085743245, -59.46198759304437, -20.007659748954865, 21.70186538498539, 58.3313842526124, 92.14771887207513, 124.27846788829885, 149.63781267082135, 160.34418743346322, 156.9672038628362, 155.27580589544817, 141.75043452049292, 110.18348482673184, 77.49474885219449, 41.987016265343726, 0.2833034955525799, -41.42622163838768, -76.37015490277572, -109.62269019977577, -131.59923904752216, -159.21959348404445, -167.67077095683558, -160.9109914514325, -151.8902022920296, -125.96705818704444, -102.29329900776088, -63.96656980859674, -33.53303112391013, 16.627671482821253, 53.82680203706004, 93.27531751700047, 122.58706992091082, 148.51021402589598, 158.65860183022428, 155.27580589544817, 156.9672038628362, 142.30842147880648, 120.3318726310601, 80.31374546450789, 48.18880881243323, 10.425878935731753, -34.6606297688355, -76.37015490277572, -108.49509155485042, -133.85443633737287, -151.8902022920296, -162.03859009635784, -164.28797502205947, -154.709198904343, -135.54583430476092, -104.54849629761163, -71.85976032307427, -32.96923180144745, 7.0430830009556615, 52.135404069672006, 85.95173868913471, 118.64047466367205, 142.30842147880648, 157.5310031852989, 159.78038811100052, 158.09480250776156, 142.30842147880648, 123.71466856583618, 86.5155380115974, 49.316407457358586, 13.244875548045162, -27.33705094096973, -69.04076371076087, -103.42089765268625, -130.4716404025968, -151.8902022920296, -160.34719212896982, -162.60238941882054, -154.14539958188033, -135.54583430476092, -104.54849629761163, -71.85976032307427, -36.91582705868622, 4.793698075254034, 51.007805424746635, 81.44134410943326, 115.82147805135864, 140.62283587556755, 154.1482072505228, 160.9079867559259, 156.40340454037351, 145.69121741358256, 120.89567195352278, 93.27531751700047, 54.95440068198541]
  out "Kulite Pressure":dbl[](array[numeric])=[67.56355890025328, 44.75208145118798, 24.0107364851398, -0.5798179133024579, -24.282652934141616, -48.873207332584016, -67.54078162144431, -81.16945698415554, -94.20510669707431, -98.3526480514498, -95.68585172446987, -85.61533026051244, -72.28134862561213, -51.54000365956394, -28.728526210498504, -3.5449461622640612, 22.82468518555516, 44.15905580139566, 67.56355890025328, 86.23113318911372, 96.59998657505243, 104.89506928380354, 103.11963052859726, 98.96845098005123, 90.97170019328152, 72.30412590442108, 49.19431653337424, 24.603762134932122, 0.3079014643006424, -23.689627284349296, -49.7645649043576, -71.39362924800902, -85.02230461072011, -95.09646426884804, -99.24400562322352, -98.6509799734312, -88.87151404311433, -73.76209365300768, -55.98587693592096, -32.87606756487413, -6.506436217054904, 20.1578888585751, 45.934494556602, 66.37750760066878, 84.15736251192597, 98.37906352442938, 106.08112058338817, 106.96883996099135, 101.04585985140945, 88.00657194432006, 74.37789658160882, 52.748832237957544, 26.677532812119725, 2.086978413677465, -22.50721417893528, -46.799436655396136, -67.54078162144431, -82.94853393353223, -88.87151404311433, -98.94567370124211, -97.17023494603578, -87.68910093770018, -74.64981303061077, -57.466621963316385, -34.35681259226955, -10.359283843619608, 15.715653776388695, 40.89923382462327, 64.00904319566997, 79.11846358577662, 96.30529284724165, 106.96883996099135, 105.78278866140677, 101.04585985140945, 90.0803426215078, 74.08320285379804, 53.934883537542184, 31.41809981628767, 6.529213495864007, -17.468315252786073, -45.0239979001898, -66.65306224384108, -81.76248263394773, -92.7243616696789, -96.5772092962436, -98.94567370124211, -91.53831037009425, -83.83625331113547, -59.83872456248553, -38.20966021883425, -12.727748248618267, 13.343551177219553, 38.825463147435535, 59.56316991931309, 77.63771855838135, 94.52621589786469, 104.00734990620043, 109.34094256016049, 101.04585985140945, 93.9331902480725, 77.93241228619213, 57.78773116410675, 31.41809981628767, 8.602984173051748, -14.50682519799509, -38.20966021883425, -60.43175021227785, -78.50266065717548, -90.35589726468024, -98.05795432363902, -99.24400562322352, -91.53831037009425, -79.9834056845709, -61.31946958988095, -38.80268586862643, -15.987570225390511, 12.455831799616313, 35.86033489847407, 58.38075681389907, 76.15697353098578, 93.34016459828018, 101.63524730703129, 108.15489126057598, 101.04585985140945, 93.04547087046926, 79.11846358577662, 59.86150184129449, 36.15866682045547, 10.975086772220752, -13.619105820391852, -38.50435394664503, -59.54039264050413, -77.90963500738316, -90.65059099249102, -97.4649286738467, -98.94567370124211, -93.31738731947122, -80.57643133436322, -64.28095964467194, -43.543252872794376, -19.247392202163034, 6.529213495864007, 32.01112546607999, 53.047164159938944, 74.97092223140115, 90.67336827130012, 101.34055357922037, 105.48809493359585, 104.89506928380354, 95.71226719744932]
  out "Zeros":dbl[](array[numeric])=[-0.0032040000000000003, -74.44292644292644, -0.6774011299435029, -0.09155, 0.0012207, 0.05065258259117547]
  out "Results Files":path[](array[path])=[path "X:/2011/Aero_Tunnel/Nick_Martin/Results_Post_Processed/New_SJ_TestR_cal_xls/3.0V/1180Hz_3.0V/RV (Check).txt", path "X:/2011/Aero_Tunnel/Nick_Martin/Results_Post_Processed/New_SJ_TestR_cal_xls/3.0V/1180Hz_3.0V/Mano (Kulite).txt", path "X:/2011/Aero_Tunnel/Nick_Martin/Results_Post_Processed/New_SJ_TestR_cal_xls/3.0V/1180Hz_3.0V/Mano (Honey).txt", path "X:/2011/Aero_Tunnel/Nick_Martin/Results_Post_Processed/New_SJ_TestR_cal_xls/3.0V/1180Hz_3.0V/RV (Vdi).txt", path "X:/2011/Aero_Tunnel/Nick_Martin/Results_Post_Processed/New_SJ_TestR_cal_xls/3.0V/1180Hz_3.0V/RV (Vin).txt", path "X:/2011/Aero_Tunnel/Nick_Martin/Results_Post_Processed/New_SJ_TestR_cal_xls/3.0V/1180Hz_3.0V/HW (Uhw).txt", path "X:/2011/Aero_Tunnel/Nick_Martin/Results_Post_Processed/New_SJ_TestR_cal_xls/3.0V/1180Hz_3.0V/Meta_data.txt"]
  out "Laser Error":bool=TRUE
  out "Hotwire Velocity":dbl[](array[numeric])=[0.14351354921948603, 0.16539807117210334, 0.16109082081380485, 0.15543415124143428, 0.14622429989298816, 0.10928162033929725, 0.0841365776141482, 0.06076766662114977, 0.048679411729960306, 0.051616349450563426, 0.06139367194659663, 0.06457002261446614, 0.08062124332076465, 0.09356245095846832, 0.09319203425942113, 0.0768208144747187, 0.0727596067504379, 0.059829369077498154, 0.03882813113184652, 0.030395372846084595, 0.02963386405351652, 0.032454086144080324, 0.04955534585005203, 0.07309500123771961, 0.0924558488702377, 0.13465994469189682, 0.16636373273765578, 0.16539807117210334, 0.1582482361042928, 0.14306753445948264, 0.11856432555283647, 0.08520376255002307, 0.06682535016611155, 0.05735230170399845, 0.045227407610996875, 0.05132217927538488, 0.06424979617706941, 0.06585670968880182, 0.08699455676529713, 0.09542382140427577, 0.08378206165048374, 0.07309500123771961, 0.06297465714489756, 0.039920917719091176, 0.02988782612838793, 0.02988782612838793, 0.03323472803352978, 0.04324884577483146, 0.07242480206963721, 0.1057390747865998, 0.12229225003588115, 0.16061531904998433, 0.1811799240887765, 0.1596664021554077, 0.1439636438370472, 0.11856432555283647, 0.08807360756579544, 0.07076212063868839, 0.0549137811991605, 0.0549137811991605, 0.05582486704572759, 0.06297465714489756, 0.07410472840402961, 0.08307484532820056, 0.09654809072899406, 0.08879784648749367, 0.07410472840402961, 0.06170872148652215, 0.03937345200193282, 0.03193627656670334, 0.02988782612838793, 0.032194919846702405, 0.04381142660353961, 0.06715020699672578, 0.09692409126281853, 0.12564721748468594, 0.15637060401358152, 0.170743992017364, 0.16491993869289245, 0.14261878968851244, 0.12734205346477945, 0.09692409126281853, 0.06747564536400422, 0.06361107429137419, 0.047230561324711845, 0.053406549314705704, 0.0661773791676738, 0.08201855256361215, 0.08952453407564889, 0.09617271256529467, 0.08916088395520194, 0.07209058670874242, 0.059829369077498154, 0.051616349450563426, 0.03507261751637898, 0.02662659294129177, 0.03560304194476849, 0.04296837017356882, 0.06361107429137419, 0.10263619212412589, 0.11815336602553328, 0.1475888573954579, 0.172216767374924, 0.16491993869289245, 0.14941781912677757, 0.12819342809614262, 0.09843432681908892, 0.0710914716795519, 0.05221084878329872, 0.05920668991357739, 0.05221084878329872, 0.06361107429137419, 0.0717569601811655, 0.09542382140427577, 0.09393348613951069, 0.09025367421921512, 0.0788847997076289, 0.063292577869209, 0.052508935451549985, 0.034020094693125835, 0.0271226594466865, 0.03349599129332029, 0.03774595367437672, 0.061079195182465865, 0.08627641326369798, 0.11570430397747819, 0.15033640233791673, 0.1697656721552543, 0.16684761558259864, 0.14941781912677757, 0.12522515425614958, 0.10888545705234481, 0.08272214399708722, 0.05582486704572759, 0.04838853897034304, 0.05102631812102672, 0.062340540841932204, 0.0761401731940124, 0.0788847997076289, 0.0924558488702377, 0.08952453407564889, 0.07750642180073175, 0.0661773791676738, 0.053106785229705106, 0.044376183521981416, 0.026134442846815806, 0.025888197366940424, 0.03693837559218241, 0.062340540841932204, 0.09061916521454463]
  out "AS Freq":dbl=29629.63 format="%.2f"
  out "Amplitude String":string="3"
  out "Frequency String":string="1180"
  out "Amp":dbl=3.0 format="%.2f"
  out "Freq":dbl=1180.0 format="%.2f"
  # "You Must have selected the \"Save Data\" option on the \nMeasurement Program for this vi to work correctly"
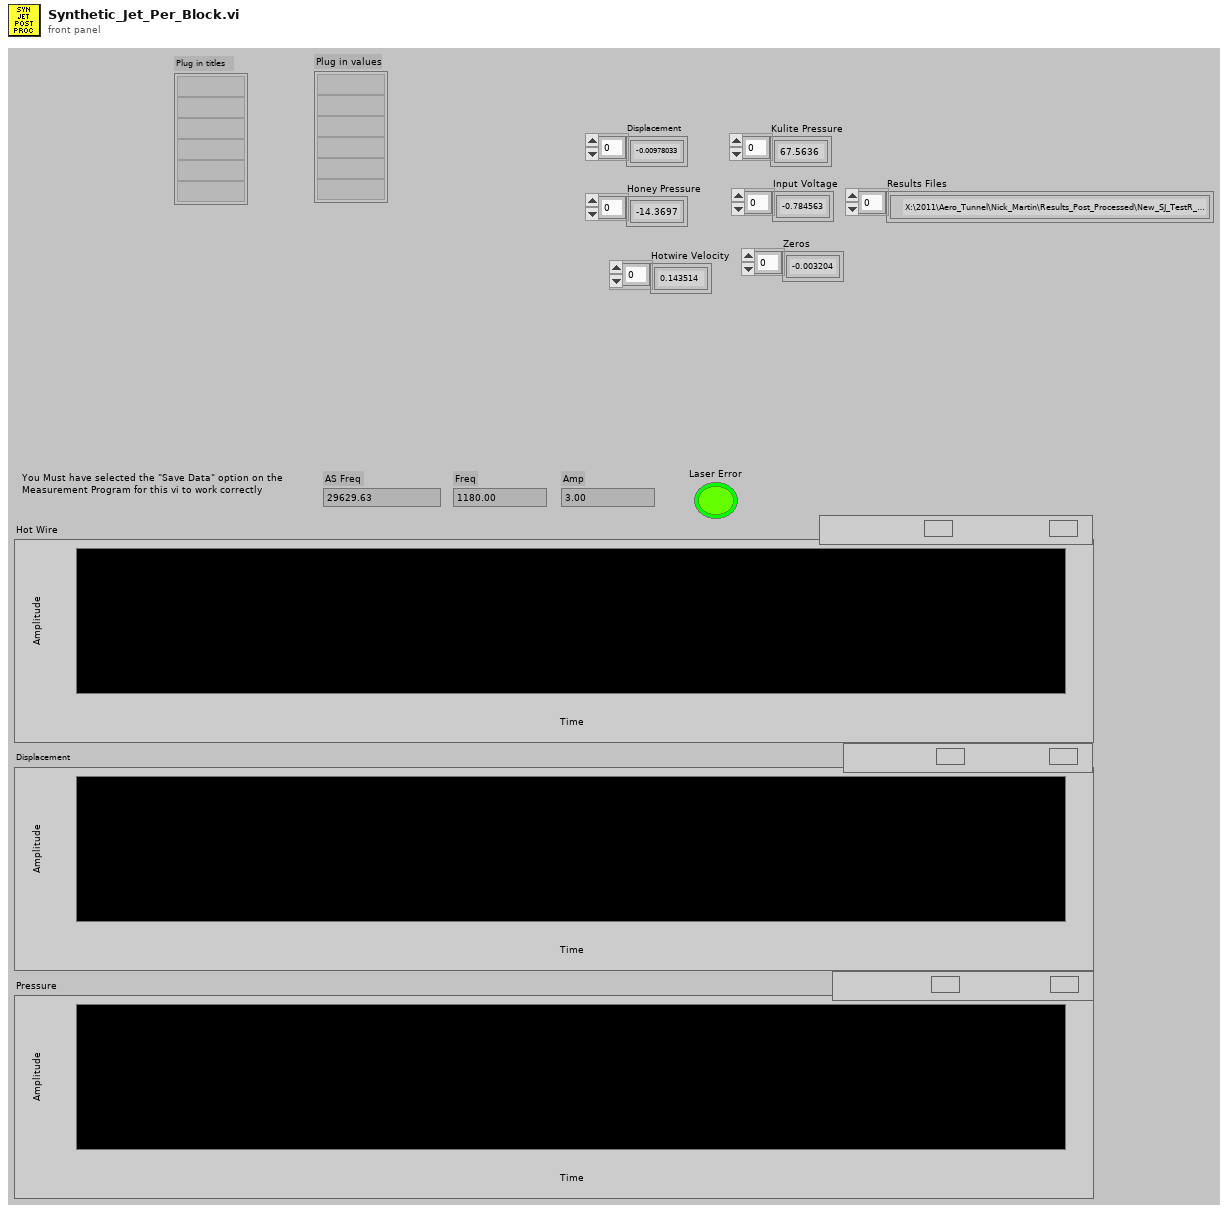
[diagram p1: front panel]
types:
  T1 = typedef "Analysis_info_cluster.ctl" = cluster{"Colour":u32, "Inst type":T2, "Inst name":string, "Symbol":string, "Code name":string, "Extra Info":string, "Inst Array":T3, "Index":i32, "Voltage Index":i32, "Extra Titles":string[], "Extra Values":string[]}
  T2 = typedef "Inst_type.ctl" = enum16{"Propeller anemometer", "Raw voltage", "Pressure Transducer", "Pitot-static tube", "Preston tube", "Hot wire", "Cross wire 1", "Cross wire 2", "Generic Linear", "Generic Polynomial", "Generic BackPoly", "Fast FID", "Thermocouple", "Cold wire", "Pulsed Wire", "LDA Vel", "LDA Tran time", "LDA Arr time"}
  T3 = typedef "Instrument_Array.ctl" = enum16{"PWA", "LDA", "Analogue"}
  T4 = cluster{"Name":string, "X":dbl, "Y":dbl, "Z":dbl}[]
  T5 = cluster{"Name":string, "X":dbl, "Y":dbl, "Z":dbl}
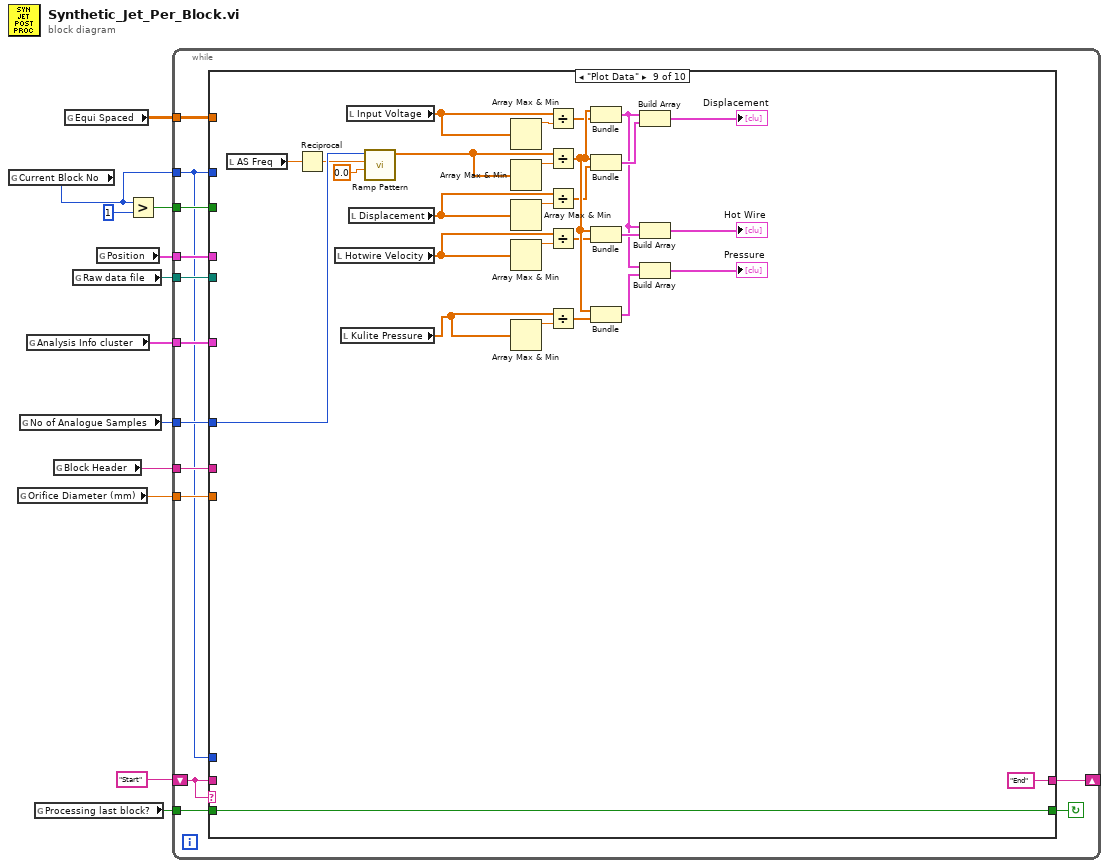
[diagram p0: block diagram]
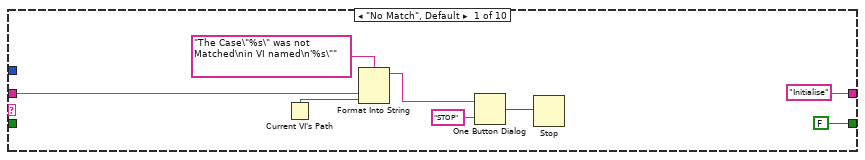
[diagram p2: hidden frame]
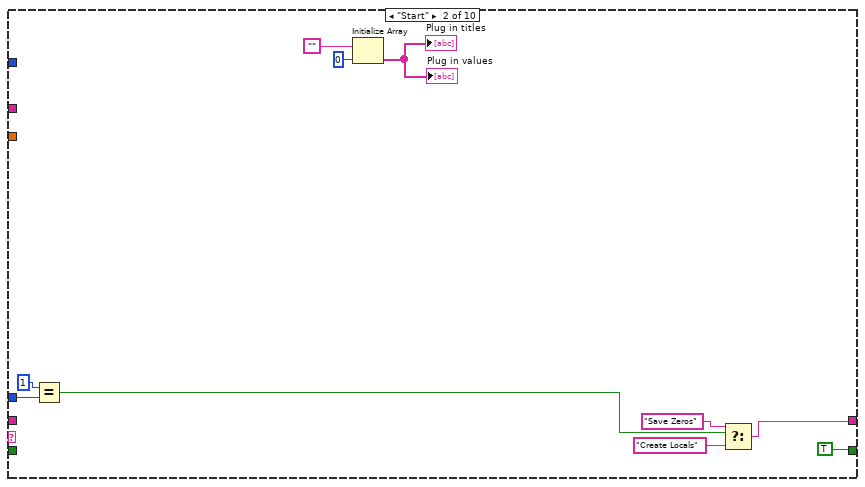
[diagram p3: hidden frame]
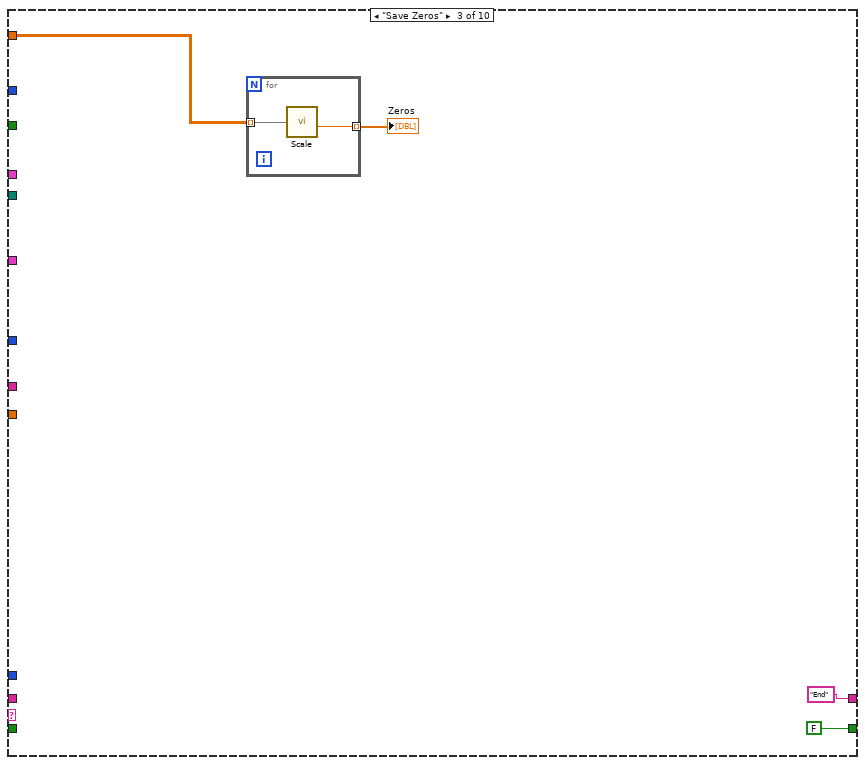
[diagram p4: hidden frame]
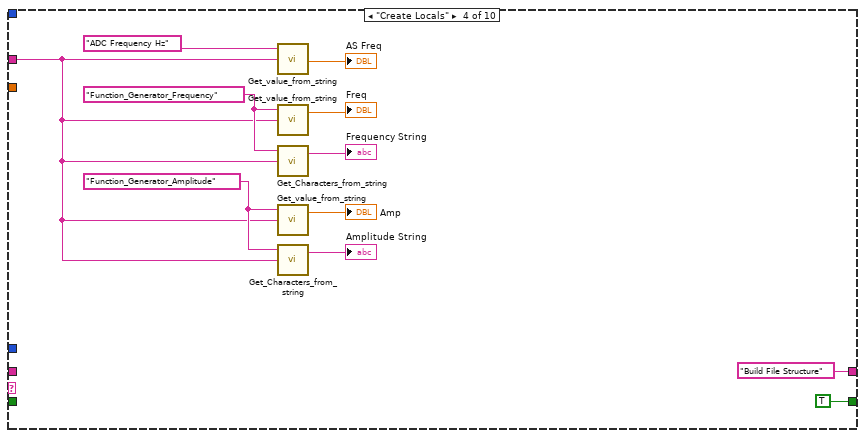
[diagram p5: hidden frame]
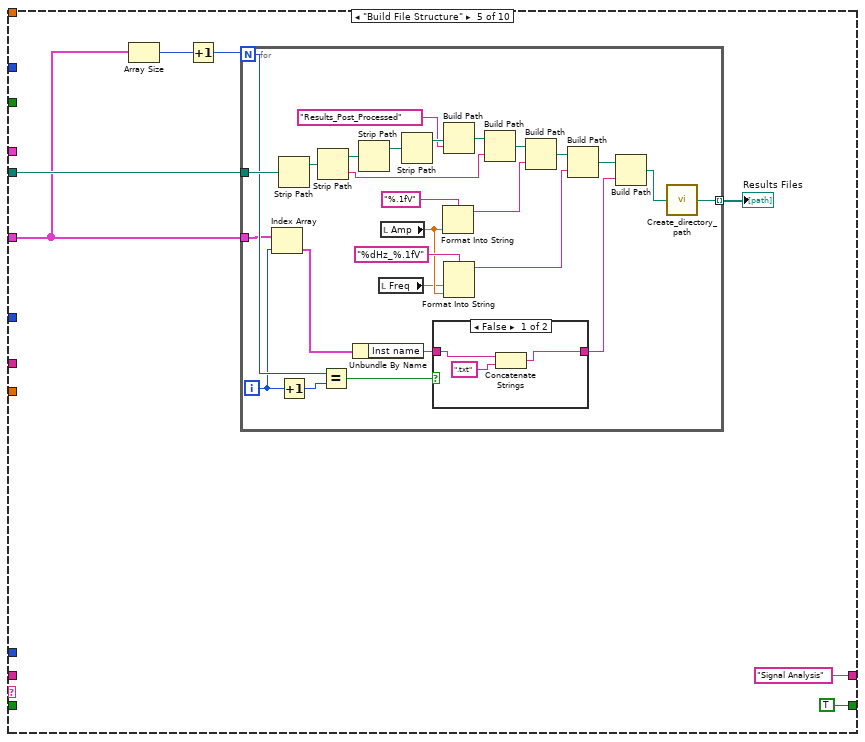
[diagram p6: hidden frame]
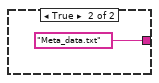
[diagram p7: hidden frame]
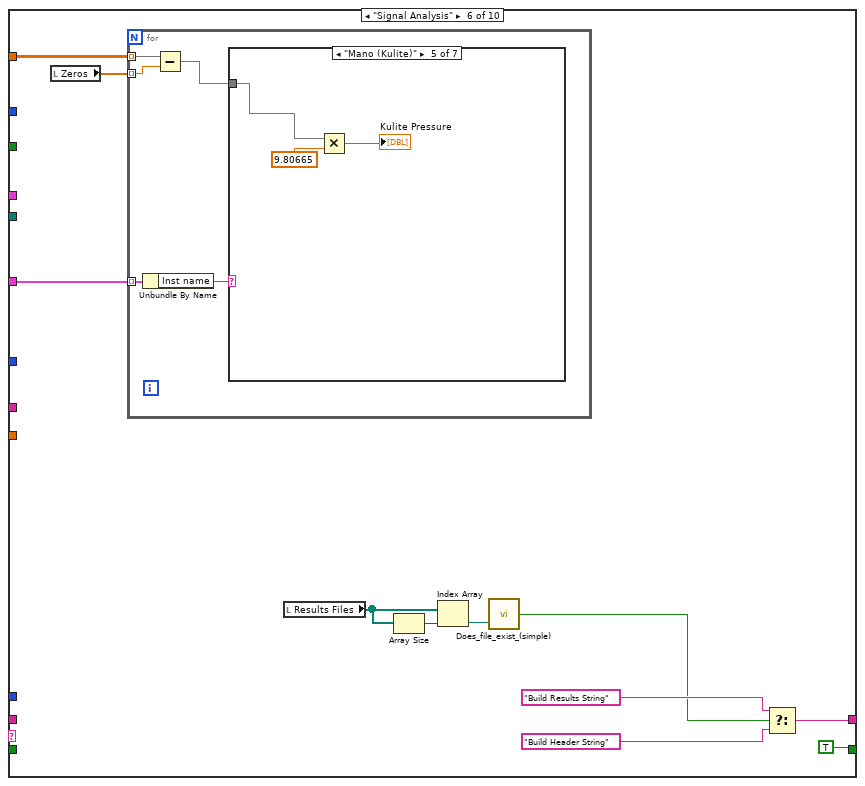
[diagram p8: hidden frame]
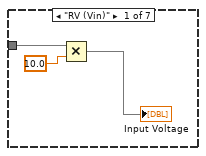
[diagram p9: hidden frame]
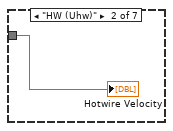
[diagram p10: hidden frame]
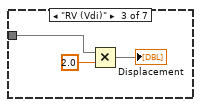
[diagram p11: hidden frame]
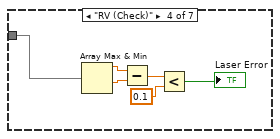
[diagram p12: hidden frame]
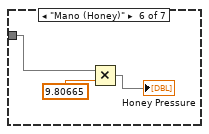
[diagram p13: hidden frame]
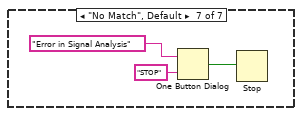
[diagram p14: hidden frame]
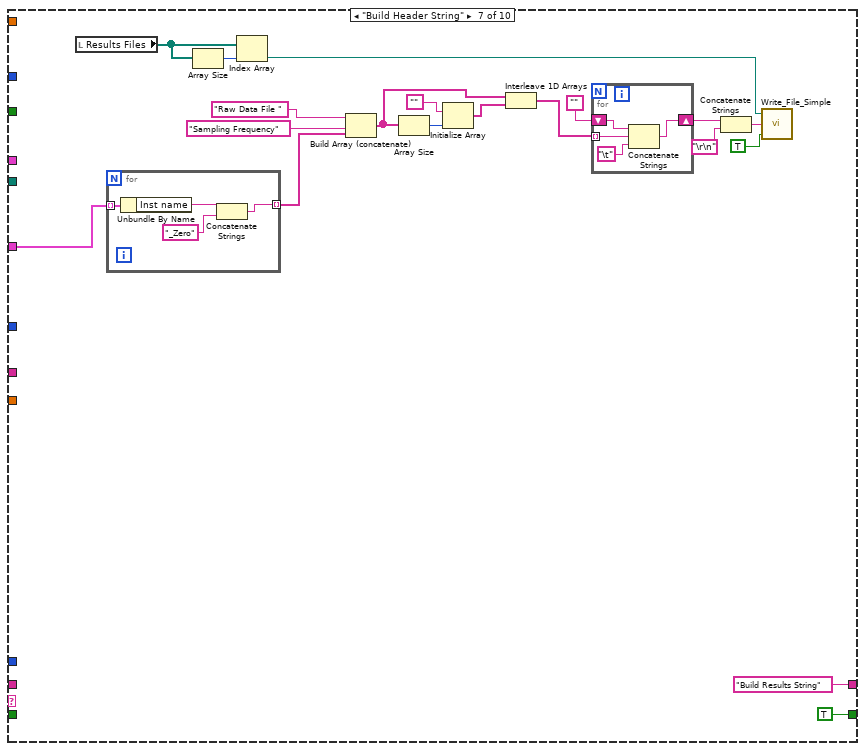
[diagram p15: hidden frame]
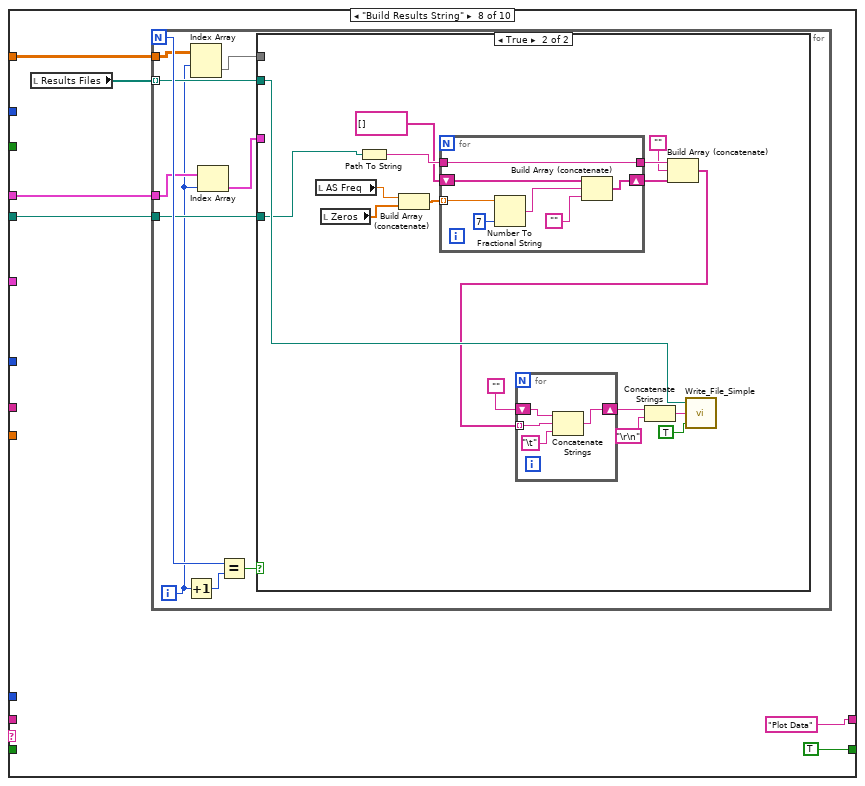
[diagram p16: hidden frame]
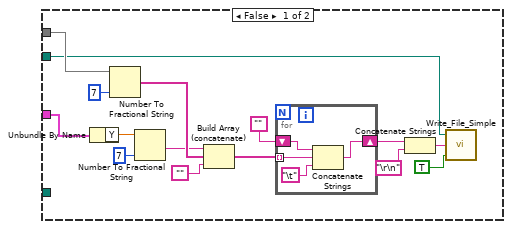
[diagram p17: hidden frame]
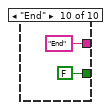
[diagram p18: hidden frame]
diagram:
  n1 = global read "Meas_global.vi" "Current Block No"() -> (w8:i32)
  n2 = global read "DataTranslation_global.vi" "Orifice Diameter (mm)"() -> (w4:dbl)
  n3 = global read "Meas_global.vi" "No of Analogue Samples"() -> (w3:i32)
  n4 = global read "Meas_global.vi" "Analysis Info cluster"() -> (w7:T1[])
  n5 = global read "Meas_global.vi" "Processing last block?"() -> (w1:bool)
  n6 = global read "Plug_in_data_global.vi" "Block Header"() -> (w5:string)
  n7 = global read "Plug_in_data_global.vi" "Equi Spaced"() -> (w6:dbl[][])
  n8 = global read "Meas_global.vi" "Raw data file"() -> (w11:path)
  n9 = global read "Meas_global.vi" "Position"() -> (w2:T4)
  n10 = Greater?(x=w8, y=1) -> (0:w9:bool)
  n11 = while {
    shift-left: "Start" -> [w25]
    shift-right: [w14] -> _
    tunnel: w11 -> [w24]
    tunnel: w9 -> [w23]
    tunnel: w8 -> [w15]
    tunnel: w7 -> [w22]
    tunnel: w6 -> [w21]
    tunnel: w5 -> [w20]
    tunnel: w4 -> [w19]
    tunnel: w3 -> [w18]
    tunnel: w2 -> [w17]
    tunnel: w1 -> [w16]
    stop <- w13 continue-if-true
    n12 = case shown="\"Plot Data\"" w25 {
      tunnel: w25 -> [w29 _ _ _ _ _ _ _ _ _]
      tunnel: w24 -> [_ _ _ _ w67 _ _ w167 _ _]
      tunnel: w23 -> [_ _ _ _ _ _ _ _ _ _]
      tunnel: w15 -> [_ _ _ _ _ _ _ _ _ _]
      tunnel: w22 -> [_ _ _ _ w62 w104 w139 _ _ _]
      tunnel: w21 -> [_ _ w47 _ _ w106 _ w168 _ _]
      tunnel: w20 -> [_ _ _ w55 _ _ _ _ _ _]
      tunnel: w19 -> [_ _ _ _ _ _ _ _ _ _]
      tunnel: w18 -> [_ _ _ _ _ _ _ _ w251 _]
      tunnel: w17 -> [_ _ _ _ _ _ _ w169 _ _]
      tunnel: w16 -> [_ _ _ _ _ _ _ _ w252 _]
      tunnel: w15 -> [_ w40 _ _ _ _ _ _ _ _]
      tunnel: ["Initialise" w35 "End" ("t") "Build File Structure" "Signal Analysis" w107 "Build Results String" "Plot Data" "End" "End"] -> w14
      tunnel: [FALSE TRUE FALSE TRUE TRUE TRUE TRUE TRUE ("Processing last block?") w252 FALSE ("Processing last block?")] -> w13
      frame "No Match", Default {
        n13 = Current VI's Path() -> (path=w28:path)
        n14 = Format Into String(format string="The Case\"%s\" was not Matched\nin VI named\n'%s\"" ("Format String"), w29, w28) -> (resulting string=w32:string)  [unwired: 2 in, 1 out]
        n15 = One Button Dialog(message=w32, button name ("OK")="STOP") -> (true=w30:bool)
        n16 = Stop(stop? (T)=w30) -> ()
      }
      frame "Start" {
        n17 = Equal?(x=1, y=w40) -> (x = y?=w38:bool)
        n18 = Initialize Array("", 0) -> (→"Plug in values" →"Plug in titles":string[])
        n19 = Select(t="Save Zeros", s=w38, f="Create Locals") -> (s? t:f=w35:string)
      }
      frame "Save Zeros" {
        (unwired) FALSE ("Processing last block?")
        (unwired) "End" ("t")
        (unwired) "End" ("t")
        (unwired) FALSE ("Processing last block?")
        n20 = for {
          tunnel: w47 -> [w49] mode=indexing
          tunnel: [w48] -> w45 mode=indexing
          n21 = call-poly <vilib>:"Scale.vi"("X"=w49) -> ("offset"=w48:dbl)  [unwired: 3 out]
        }
        "Zeros" <- w45
      }
      frame "Create Locals" {
        w57 = "Function_Generator_Amplitude" ("Variable name")
        w58 = "Function_Generator_Frequency" ("Variable name")
        n22 = call "Get_value_from_string.vi"("Input string"=w55, "Variable name"="ADC Frequency Hz") -> ("Value"=→"AS Freq":dbl)  [unwired: 1 in, 1 out]
        n23 = call "Get_value_from_string.vi"("Input string"=w55, "Variable name"=w58) -> ("Value"=→"Freq":dbl)  [unwired: 1 in, 1 out]
        n24 = call "Get_Characters_from_string.vi"("Input string"=w55, "Variable name"=w58) -> ("Value"=→"Frequency String":string)  [unwired: 1 in, 1 out]
        n25 = call "Get_value_from_string.vi"("Input string"=w55, "Variable name"=w57) -> ("Value"=→"Amp":dbl)  [unwired: 1 in, 1 out]
        n26 = call "Get_Characters_from_string.vi"("Input string"=w55, "Variable name"=w57) -> ("Value"=→"Amplitude String":string)  [unwired: 1 in, 1 out]
      }
      frame "Build File Structure" {
        n27 = Array Size(array=w62) -> (size(s)=w61:i32)
        n28 = Increment(x=w61) -> (x+1=w65:i32)
        n29 = for {
          N: w65 -> [w76]
          tunnel: w67 -> [w85]
          tunnel: [w84] -> w66 mode=indexing
          tunnel: w62 -> [w70]
          i -> [w68]
          n30 = Index Array(array=w70, index=w68) -> (element=w69:T1)
          n31 = Strip Path(path=w85) -> (stripped path=w94:path)  [unwired: 1 out]
          n32 = Increment(x=w68) -> (x+1=w71:i32)
          n33 = Strip Path(path=w94) -> (stripped path=w92:path, name=w88:string)
          n34 = Equal?(x=w76, y=w71) -> (x = y?=w74:bool)
          n35 = Unbundle By Name(w69) -> ("Inst name"=w73:string)
          n36 = Strip Path(path=w92) -> (stripped path=w93:path)  [unwired: 1 out]
          n37 = local read "Freq"() -> (w79:dbl)
          n38 = local read "Amp"() -> (w80:dbl)
          n39 = Strip Path(path=w93) -> (stripped path=w91:path)  [unwired: 1 out]
          n40 = case shown="False" w74 {
            tunnel: w73 -> [w97 _]
            tunnel: [w95 "Meta_data.txt"] -> w72
            frame False {
              n41 = Concatenate Strings(w97, ".txt" ("string")) -> (w95:string)
            }
            frame True {
            }
          }
          n42 = Format Into String(format string="%.1fV", w80) -> (resulting string=w82:string)  [unwired: 2 in, 1 out]
          n43 = Build Path(base path=w91, name or relative path="Results_Post_Processed") -> (appended path=w89:path)
          n44 = Format Into String(format string="%dHz_%.1fV", w79, w80) -> (resulting string=w78:string)  [unwired: 2 in, 1 out]
          n45 = Build Path(base path=w89, name or relative path=w88) -> (appended path=w87:path)
          n46 = Build Path(base path=w87, name or relative path=w82) -> (appended path=w86:path)
          n47 = Build Path(base path=w86, name or relative path=w78) -> (appended path=w77:path)
          n48 = Build Path(base path=w77, name or relative path=w72) -> (appended path=w75:path)
          n49 = call "Create_directory_path.vi"("Path name"=w75) -> ("Path name Out"=w84:path)
        }
        "Results Files" <- w66
      }
      frame "Signal Analysis" {
        n50 = local read "Zeros"() -> (w105:dbl[])
        n51 = for {
          tunnel: w106 -> [w114] mode=indexing
          tunnel: w105 -> [w113] mode=indexing
          tunnel: w104 -> [w112] mode=indexing
          n52 = Unbundle By Name(w112) -> ("Inst name"=w110:string)
          n53 = Subtract(x=w114, y=w113) -> (x-y=w111:dbl[])
          n54 = case shown="\"Mano (Kulite)\"" w110 {
            tunnel: w111 -> [w117 w118 w120 w123 w130 w132 _]
            frame "RV (Vin)" {
              n55 = Multiply(x=w117, y=10.0) -> (x*y=→"Input Voltage":dbl[])
            }
            frame "HW (Uhw)" {
              "Hotwire Velocity" <- w118
            }
            frame "RV (Vdi)" {
              n56 = Multiply(x=w120, y=2.0) -> (x*y=→"Displacement":dbl[])
            }
            frame "RV (Check)" {
              n57 = Array Max & Min(array=w123) -> (max value=w124:dbl, min value=w125:dbl)  [unwired: 2 out]
              n58 = Subtract(x=w124, y=w125) -> (x-y=w126:dbl)
              n59 = Less?(x=w126, y=0.1) -> (x < y?=→"Laser Error":bool)
            }
            frame "Mano (Kulite)" {
              n60 = Multiply(x=w130, y=9.80665) -> (x*y=→"Kulite Pressure":dbl[])
            }
            frame "Mano (Honey)" {
              n61 = Multiply(x=w132, y=9.80665) -> (x*y=→"Honey Pressure":dbl[])
            }
            frame "No Match", Default {
              n62 = One Button Dialog(message="Error in Signal Analysis", button name ("OK")="STOP") -> (true=w135:bool)
              n63 = Stop(stop? (T)=w135) -> ()
            }
          }
        }
        n64 = local read "Results Files"() -> (w101:path[])
        n65 = Array Size(array=w101) -> (size(s)=w102:i32)
        n66 = Index Array(array=w101, index=w102) -> (element=w100:path)
        n67 = call "Does_file_exist_(simple).vi"("Pathname"=w100) -> ("exists?"=w99:bool)
        n68 = Select(t="Build Results String", s=w99, f="Build Header String") -> (s? t:f=w107:string)
      }
      frame "Build Header String" {
        n69 = local read "Results Files"() -> (w141:path[])
        n70 = for {
          tunnel: w139 -> [w159] mode=indexing
          tunnel: [w157] -> w138 mode=indexing
          n71 = Unbundle By Name(w159) -> ("Inst name"=w158:string)
          n72 = Concatenate Strings(w158, "_Zero" ("string")) -> (w157:string)
        }
        n73 = Array Size(array=w141) -> (size(s)=w142:i32)
        n74 = Index Array(array=w141, index=w142) -> (element=w140:path)
        n75 = Build Array (concatenate)("Raw Data File ", "Sampling Frequency" ("element"), w138) -> (w153:string[])
        n76 = Array Size(array=w153) -> (size(s)=w152:i32)
        n77 = Initialize Array("", w152) -> (w154:string[])
        n78 = Interleave 1D Arrays(w153, w154) -> (w145:string[])
        n79 = for {
          shift-right: [w162] -> w149
          shift-left: "" -> [w163]
          tunnel: w145 -> [w161] mode=indexing
          n80 = Concatenate Strings(w163, w161, "\t") -> (w162:string)
        }
        n81 = Concatenate Strings(w149, "\r\n") -> (w150:string)
        n82 = call "Write_File_Simple.vi"("append to file? (new file:F)"=TRUE, "character string"=w150, "file path"=w140) -> ()  [unwired: 2 out]
      }
      frame "Build Results String" {
        n83 = local read "Results Files"() -> (w164:path[])
        n84 = for {
          N -> [w179]
          tunnel: w164 -> [w177] mode=indexing
          tunnel: w168 -> [w174]
          tunnel: w169 -> [w172]
          tunnel: w167 -> [w175]
          i -> [w171]
          n85 = Increment(x=w171) -> (x+1=w176:i32)
          n86 = Index Array(array=w174, index (row)=w171) -> (element=w173:dbl[])  [unwired: 1 in]
          n87 = Index Array(array=w172, index=w171) -> (element=w170:T5)
          n88 = Equal?(x=w179, y=w176) -> (x = y?=w178:bool)
          n89 = case shown="True" w178 {
            tunnel: w173 -> [w188 _]
            tunnel: w177 -> [w180 w203]
            tunnel: w170 -> [w187 _]
            tunnel: w175 -> [_ w201]
            frame False {
              n90 = Unbundle By Name(w187) -> ("Y"=w190:dbl)
              n91 = Number To Fractional String(number=w188, precision (6)=i16 7) -> (F-format string=w194:string[])  [unwired: 2 in]
              n92 = Number To Fractional String(number=w190, precision (6)=i16 7) -> (F-format string=w192:string)  [unwired: 2 in]
              n93 = Build Array (concatenate)(w192, w194, "") -> (w181:string[])
              n94 = for {
                shift-right: [w197] -> w185
                shift-left: "" -> [w198]
                tunnel: w181 -> [w196] mode=indexing
                n95 = Concatenate Strings(w198, w196, "\t") -> (w197:string)
              }
              n96 = Concatenate Strings(w185, "\r\n") -> (w186:string)
              n97 = call "Write_File_Simple.vi"("append to file? (new file:F)"=TRUE, "character string"=w186, "file path"=w180) -> ()  [unwired: 2 out]
            }
            frame True {
              n98 = local read "AS Freq"() -> (w200:dbl)
              n99 = local read "Zeros"() -> (w199:dbl[])
              n100 = Path To String(path=w201) -> (string=w213:string)
              n101 = Build Array (concatenate)(w200, w199) -> (w214:dbl[])
              n102 = for {
                tunnel: w214 -> [w224] mode=indexing
                tunnel: w213 -> [w219]
                shift-right: [w220] -> w211
                shift-left: string[] [] -> [w221]
                tunnel: [w219] -> w212
                n103 = Number To Fractional String(number=w224, precision (6)=i16 7) -> (F-format string=w222:string)  [unwired: 2 in]
                n104 = Build Array (concatenate)(w221, w222, "") -> (w220:string[])
              }
              n105 = Build Array (concatenate)(w212, "", w211) -> (w202:string[])
              n106 = for {
                shift-right: [w217] -> w205
                shift-left: "" -> [w218]
                tunnel: w202 -> [w216] mode=indexing
                n107 = Concatenate Strings(w218, w216, "\t") -> (w217:string)
              }
              n108 = Concatenate Strings(w205, "\r\n") -> (w204:string)
              n109 = call "Write_File_Simple.vi"("append to file? (new file:F)"=TRUE, "character string"=w204, "file path"=w203) -> ()  [unwired: 2 out]
            }
          }
        }
      }
      frame "Plot Data" {
        n110 = local read "AS Freq"() -> (w249:dbl)
        n111 = Reciprocal(x=w249) -> (1/x=w248:dbl)
        n112 = local read "Hotwire Velocity"() -> (w227:dbl[])
        n113 = local read "Kulite Pressure"() -> (w226:dbl[])
        n114 = local read "Input Voltage"() -> (w229:dbl[])
        n115 = local read "Displacement"() -> (w228:dbl[])
        n116 = call-poly <vilib>:"Ramp Pattern.vi"("start"=0.0, "end"=w248, "samples"=w251) -> ("Ramp Pattern"=w239:dbl[])  [unwired: 7 in, 1 out]
        n117 = Array Max & Min(array=w229) -> (max value=w237:dbl)  [unwired: 3 out]
        n118 = Array Max & Min(array=w239) -> (max value=w240:dbl)  [unwired: 3 out]
        n119 = Array Max & Min(array=w228) -> (max value=w233:dbl)  [unwired: 3 out]
        n120 = Array Max & Min(array=w227) -> (max value=w235:dbl)  [unwired: 3 out]
        n121 = Array Max & Min(array=w226) -> (max value=w231:dbl)  [unwired: 3 out]
        n122 = Divide(x=w229, y=w237) -> (x/y=w236:dbl[])
        n123 = Divide(x=w239, y=w240) -> (x/y=w238:dbl[])
        n124 = Divide(x=w228, y=w233) -> (x/y=w232:dbl[])
        n125 = Divide(x=w227, y=w235) -> (x/y=w234:dbl[])
        n126 = Divide(x=w226, y=w231) -> (x/y=w230:dbl[])
        n127 = Bundle(w238, w236) -> (w245:cluster{dbl[], dbl[]})  [unwired: 1 in]
        n128 = Bundle(w238, w232) -> (w246:cluster{dbl[], dbl[]})  [unwired: 1 in]
        n129 = Bundle(w238, w234) -> (w247:cluster{dbl[], dbl[]})  [unwired: 1 in]
        n130 = Bundle(w238, w230) -> (w244:cluster{dbl[], dbl[]})  [unwired: 1 in]
        n131 = Build Array(w245, w246) -> (→"Displacement":cluster{dbl[], dbl[]}[])
        n132 = Build Array(w245, w247) -> (→"Hot Wire":cluster{dbl[], dbl[]}[])
        n133 = Build Array(w245, w244) -> (→"Pressure":cluster{dbl[], dbl[]}[])
      }
      frame "End" {
      }
    }
  }
